vi "DblMonoPMDCurrentScanSM correction.vi"() -> ()   [LabVIEW 2010]
uses:
  <vilib>/DAQmx/write.llb/DAQmx Write (Analog DBL 1Chan 1Samp).vi
  <vilib>/DAQmx/read.llb/DAQmx Read (Analog 1D DBL 1Chan NSamp).vi
  <vilib>/DAQmx/read.llb/DAQmx Read (Analog 1D DBL NChan 1Samp).vi
  <vilib>/DAQmx/write.llb/DAQmx Write (Analog 2D DBL NChan NSamp).vi
  <vilib>/DAQmx/create/channels.llb/DAQmx Create Channel (AO-Voltage-Basic).vi
  <vilib>/DAQmx/create/channels.llb/DAQmx Create Channel (AI-Voltage-Basic).vi
  <vilib>/daqmx/miscellaneous.llb/DAQmx Fill In Error Info.vi
  <vilib>/DAQmx/configure/timing.llb/DAQmx Timing (Sample Clock).vi
  <vilib>/Utility/file.llb/Write To Spreadsheet File (DBL).vi
  <vilib>/Analysis/NI_AALBase.lvlib
panel:
  out "element 2":dbl=0.021735275146704158
  out "element":dbl=0.029564787036695163
  out "number of samples written per channel":u32=999
  out "Waveform Chart  Y":dbl[](graph)=[0.022057757713531734, 0.02205806778326472, 0.022058377852997708, 0.022058687922730698, 0.022058997992463684, 0.02205930806219667, 0.022059618131929658, 0.022059928201662644, 0.022060238271395635, 0.02206054834112862, 0.022060858410861608, 0.022061168480594594, 0.02206147855032758, 0.02206178862006057, 0.022062098689793558, 0.022062408759526544, 0.02206271882925953, 0.022063028898992518, 0.022063338968725504, 0.022063649038458494, 0.02206395910819148, 0.022064269177924468, 0.022064579247657454, 0.02206488931739044, 0.02206519938712343, 0.022065509456856418, 0.022065819526589404, 0.02206612959632239, 0.022066439666055378, 0.022066749735788368, 0.022067059805521354, 0.02206736987525434, 0.022067679944987328, 0.022067990014720314, 0.022068300084453304, 0.02206861015418629, 0.022068920223919278, 0.022069230293652264, 0.02206954036338525, 0.022069850433118238, 0.022070160502851228, 0.022070470572584214, 0.0220707806423172, 0.022071090712050188, 0.022071400781783174, 0.022071710851516164, 0.02207202092124915, 0.022072330990982138, 0.022072641060715124, 0.02207295113044811, 0.0220732612001811, 0.022073571269914088, 0.022073881339647074, 0.02207419140938006, 0.022074501479113048, 0.022074811548846038, 0.022075121618579024, 0.02207543168831201, 0.022075741758044998, 0.022076051827777984, 0.022076361897510974, 0.02207667196724396, 0.022076982036976948, 0.022077292106709934, 0.02207760217644292, 0.022077912246175908, 0.022078222315908898, 0.022078532385641884, 0.02207884245537487, 0.022079152525107858, 0.022079462594840844, 0.022079772664573834, 0.02208008273430682, 0.022080392804039808, 0.022080702873772794, 0.02208101294350578, 0.02208132301323877, 0.022081633082971758, 0.022081943152704744, 0.02208225322243773, 0.022082563292170718, 0.022082873361903708, 0.022083183431636694, 0.02208349350136968, 0.022083803571102668, 0.022084113640835654, 0.022084423710568644, 0.02208473378030163, 0.022085043850034618, 0.022085353919767604, 0.02208566398950059, 0.022085974059233578, 0.022086284128966568, 0.022086594198699554, 0.02208690426843254, 0.022087214338165528, 0.022087524407898514, 0.022087834477631504, 0.02208814454736449, 0.022088454617097478, 0.022088764686830464, 0.02208907475656345, 0.02208938482629644, 0.022089694896029428, 0.022090004965762414, 0.0220903150354954, 0.022090625105228388, 0.022090935174961378, 0.022091245244694364, 0.02209155531442735, 0.022091865384160338, 0.022092175453893324, 0.022092485523626314, 0.0220927955933593, 0.022093105663092288, 0.022093415732825274, 0.02209372580255826, 0.022094035872291248, 0.022094345942024238, 0.022094656011757224, 0.02209496608149021, 0.022095276151223198, 0.022095586220956184, 0.022095896290689174, 0.02209620636042216, 0.022096516430155148, 0.022096826499888134, 0.02209713656962112, 0.02209744663935411, 0.022097756709087098, 0.022098066778820084, 0.02209837684855307, 0.022098686918286058, 0.022098996988019048, 0.022099307057752034, 0.02209961712748502, 0.022099927197218008, 0.022100237266950994, 0.022100547336683984, 0.02210085740641697, 0.022101167476149958, 0.022101477545882944, 0.02210178761561593, 0.022102097685348918, 0.022102407755081908, 0.022102717824814894, 0.02210302789454788, 0.022103337964280868, 0.022103648034013854, 0.022103958103746844, 0.02210426817347983, 0.022104578243212818, 0.022104888312945804, 0.02210519838267879, 0.02210550845241178, 0.022105818522144768, 0.022106128591877754, 0.02210643866161074, 0.022106748731343728, 0.022107058801076718, 0.022107368870809704, 0.02210767894054269, 0.022107989010275678, 0.022108299080008664, 0.02210860914974165, 0.02210891921947464, 0.022109229289207628, 0.022109539358940614, 0.0221098494286736, 0.022110159498406588, 0.022110469568139578, 0.022110779637872564, 0.02211108970760555, 0.022111399777338538, 0.022111709847071524, 0.022112019916804514, 0.0221123299865375, 0.022112640056270488, 0.022112950126003474, 0.02211326019573646, 0.02211357026546945, 0.022113880335202438, 0.022114190404935424, 0.02211450047466841, 0.022114810544401398, 0.022115120614134388, 0.022115430683867374, 0.02211574075360036, 0.022116050823333348, 0.022116360893066334, 0.02211667096279932, 0.02211698103253231, 0.022117291102265298, 0.022117601171998284, 0.02211791124173127, 0.022118221311464258, 0.022118531381197248, 0.022118841450930234, 0.02211915152066322, 0.022119461590396208, 0.022119771660129194, 0.022120081729862184, 0.02212039179959517, 0.022120701869328158, 0.022121011939061144, 0.02212132200879413, 0.02212163207852712, 0.022121942148260108, 0.022122252217993094, 0.02212256228772608, 0.022122872357459068, 0.022123182427192058, 0.022123492496925044, 0.02212380256665803, 0.022124112636391018, 0.022124422706124004, 0.02212473277585699, 0.02212504284558998, 0.022125352915322968, 0.022125662985055954, 0.02212597305478894, 0.022126283124521928, 0.022126593194254918, 0.022126903263987904, 0.02212721333372089, 0.022127523403453878, 0.022127833473186864, 0.022128143542919854, 0.02212845361265284, 0.022128763682385828, 0.022129073752118814, 0.0221293838218518, 0.02212969389158479, 0.022130003961317778, 0.022130314031050764, 0.02213062410078375, 0.022130934170516738, 0.022131244240249728, 0.022131554309982714, 0.0221318643797157, 0.022132174449448688, 0.022132484519181674, 0.02213279458891466, 0.02213310465864765, 0.022133414728380638, 0.022133724798113624, 0.02213403486784661, 0.022134344937579598, 0.022134655007312588, 0.022134965077045574, 0.02213527514677856, 0.022135585216511548, 0.022135895286244534, 0.022136205355977524, 0.02213651542571051, 0.022136825495443498, 0.022137135565176484, 0.02213744563490947, 0.02213775570464246, 0.022138065774375448, 0.022138375844108434, 0.02213868591384142, 0.022138995983574408, 0.022139306053307398, 0.022139616123040384, 0.02213992619277337, 0.022140236262506358, 0.022140546332239344, 0.02214085640197233, 0.02214116647170532, 0.022141476541438308, 0.022141786611171294, 0.02214209668090428, 0.022142406750637268, 0.022142716820370258, 0.022143026890103244, 0.02214333695983623, 0.022143647029569218, 0.022143957099302204, 0.022144267169035194, 0.02214457723876818, 0.022144887308501168, 0.022145197378234154, 0.02214550744796714, 0.02214581751770013, 0.022146127587433118, 0.022146437657166104, 0.02214674772689909, 0.022147057796632078, 0.022147367866365064, 0.022147677936098054, 0.02214798800583104, 0.022148298075564028, 0.022148608145297014, 0.02214891821503, 0.02214922828476299, 0.022149538354495978, 0.022149848424228964, 0.02215015849396195, 0.022150468563694937, 0.022150778633427928, 0.022151088703160914, 0.0221513987728939, 0.022151708842626888, 0.022152018912359874, 0.022152328982092864, 0.02215263905182585, 0.022152949121558838, 0.022153259191291824, 0.02215356926102481, 0.0221538793307578, 0.022154189400490788, 0.022154499470223774, 0.02215480953995676, 0.022155119609689748, 0.022155429679422734, 0.022155739749155724, 0.02215604981888871, 0.022156359888621698, 0.022156669958354684, 0.02215698002808767, 0.02215729009782066, 0.022157600167553648, 0.022157910237286634, 0.02215822030701962, 0.022158530376752607, 0.022158840446485598, 0.022159150516218584, 0.02215946058595157, 0.022159770655684558, 0.022160080725417544, 0.022160390795150534, 0.02216070086488352, 0.022161010934616508, 0.022161321004349494, 0.02216163107408248, 0.02216194114381547, 0.022162251213548458, 0.022162561283281444, 0.02216287135301443, 0.022163181422747417, 0.022163491492480404, 0.022163801562213394, 0.02216411163194638, 0.022164421701679368, 0.022164731771412354, 0.02216504184114534, 0.02216535191087833, 0.022165661980611318, 0.022165972050344304, 0.02216628212007729, 0.022166592189810277, 0.022166902259543268, 0.022167212329276254, 0.02216752239900924, 0.022167832468742227, 0.022168142538475214, 0.022168452608208204, 0.02216876267794119, 0.022169072747674178, 0.022169382817407164, 0.02216969288714015, 0.02217000295687314, 0.022170313026606128, 0.022170623096339114, 0.0221709331660721, 0.022171243235805087, 0.022171553305538074, 0.022171863375271064, 0.02217217344500405, 0.022172483514737037, 0.022172793584470024, 0.02217310365420301, 0.022173413723936, 0.022173723793668988, 0.022174033863401974, 0.02217434393313496, 0.022174654002867947, 0.022174964072600938, 0.022175274142333924, 0.02217558421206691, 0.022175894281799897, 0.022176204351532884, 0.022176514421265874, 0.02217682449099886, 0.022177134560731847, 0.022177444630464834, 0.02217775470019782, 0.02217806476993081, 0.022178374839663798, 0.022178684909396784, 0.02217899497912977, 0.022179305048862757, 0.022179615118595744, 0.022179925188328734, 0.02218023525806172, 0.022180545327794707, 0.022180855397527694, 0.02218116546726068, 0.02218147553699367, 0.022181785606726658, 0.022182095676459644, 0.02218240574619263, 0.022182715815925617, 0.022183025885658608, 0.022183335955391594, 0.02218364602512458, 0.022183956094857567, 0.022184266164590554, 0.022184576234323544, 0.02218488630405653, 0.022185196373789517, 0.022185506443522504, 0.02218581651325549, 0.022186126582988477, 0.022186436652721468, 0.022186746722454454, 0.02218705679218744, 0.022187366861920427, 0.022187676931653414, 0.022187987001386404, 0.02218829707111939, 0.022188607140852377, 0.022188917210585364, 0.02218922728031835, 0.02218953735005134, 0.022189847419784327, 0.022190157489517314, 0.0221904675592503, 0.022190777628983287, 0.022191087698716278, 0.022191397768449264, 0.02219170783818225, 0.022192017907915237, 0.022192327977648224, 0.022192638047381214, 0.0221929481171142, 0.022193258186847187, 0.022193568256580174, 0.02219387832631316, 0.022194188396046147, 0.022194498465779137, 0.022194808535512124, 0.02219511860524511, 0.022195428674978097, 0.022195738744711084, 0.022196048814444074, 0.02219635888417706, 0.022196668953910047, 0.022196979023643034, 0.02219728909337602, 0.02219759916310901, 0.022197909232841997, 0.022198219302574984, 0.02219852937230797, 0.022198839442040957, 0.022199149511773947, 0.022199459581506934, 0.02219976965123992, 0.022200079720972907, 0.022200389790705894, 0.022200699860438884, 0.02220100993017187, 0.022201319999904857, 0.022201630069637844, 0.02220194013937083, 0.022202250209103817, 0.022202560278836807, 0.022202870348569794, 0.02220318041830278, 0.022203490488035767, 0.022203800557768754, 0.022204110627501744, 0.02220442069723473, 0.022204730766967717, 0.022205040836700704, 0.02220535090643369, 0.02220566097616668, 0.022205971045899667, 0.022206281115632654, 0.02220659118536564, 0.022206901255098627, 0.022207211324831617, 0.022207521394564604, 0.02220783146429759, 0.022208141534030577, 0.022208451603763564, 0.022208761673496554, 0.02220907174322954, 0.022209381812962527, 0.022209691882695514, 0.0222100019524285, 0.022210312022161487, 0.022210622091894477, 0.022210932161627464, 0.02221124223136045, 0.022211552301093437, 0.022211862370826424, 0.022212172440559414, 0.0222124825102924, 0.022212792580025387, 0.022213102649758374, 0.02221341271949136, 0.02221372278922435, 0.022214032858957337, 0.022214342928690324, 0.02221465299842331, 0.022214963068156297, 0.022215273137889287, 0.022215583207622274, 0.02221589327735526, 0.022216203347088247, 0.022216513416821234, 0.02221682348655422, 0.02221713355628721, 0.022217443626020197, 0.022217753695753184, 0.02221806376548617, 0.022218373835219157, 0.022218683904952147, 0.022218993974685134, 0.02221930404441812, 0.022219614114151107, 0.022219924183884094, 0.022220234253617084, 0.02222054432335007, 0.022220854393083057, 0.022221164462816044, 0.02222147453254903, 0.02222178460228202, 0.022222094672015007, 0.022222404741747994, 0.02222271481148098, 0.022223024881213967, 0.022223334950946957, 0.022223645020679944, 0.02222395509041293, 0.022224265160145917, 0.022224575229878904, 0.02222488529961189, 0.02222519536934488, 0.022225505439077867, 0.022225815508810854, 0.02222612557854384, 0.022226435648276827, 0.022226745718009817, 0.022227055787742804, 0.02222736585747579, 0.022227675927208777, 0.022227985996941764, 0.022228296066674754, 0.02222860613640774, 0.022228916206140727, 0.022229226275873714, 0.0222295363456067, 0.02222984641533969, 0.022230156485072677, 0.022230466554805664, 0.02223077662453865, 0.022231086694271637, 0.022231396764004627, 0.022231706833737614, 0.0222320169034706, 0.022232326973203587, 0.022232637042936574, 0.02223294711266956, 0.02223325718240255, 0.022233567252135537, 0.022233877321868524, 0.02223418739160151, 0.022234497461334497, 0.022234807531067487, 0.022235117600800474, 0.02223542767053346, 0.022235737740266447, 0.022236047809999434, 0.022236357879732424, 0.02223666794946541, 0.022236978019198397, 0.022237288088931384, 0.02223759815866437, 0.02223790822839736, 0.022238218298130347, 0.022238528367863334, 0.02223883843759632, 0.022239148507329307, 0.022239458577062297, 0.022239768646795284, 0.02224007871652827, 0.022240388786261257, 0.022240698855994244, 0.02224100892572723, 0.02224131899546022, 0.022241629065193207, 0.022241939134926194, 0.02224224920465918, 0.022242559274392167, 0.022242869344125157, 0.022243179413858144, 0.02224348948359113, 0.022243799553324117, 0.022244109623057104, 0.022244419692790094, 0.02224472976252308, 0.022245039832256067, 0.022245349901989054, 0.02224565997172204, 0.02224597004145503, 0.022246280111188017, 0.022246590180921004, 0.02224690025065399, 0.022247210320386977, 0.022247520390119967, 0.022247830459852954, 0.02224814052958594, 0.022248450599318927, 0.022248760669051914, 0.0222490707387849, 0.02224938080851789, 0.022249690878250877, 0.022250000947983864, 0.02225031101771685, 0.022250621087449837, 0.022250931157182827, 0.022251241226915814, 0.0222515512966488, 0.022251861366381787, 0.022252171436114774, 0.022252481505847764, 0.02225279157558075, 0.022253101645313737, 0.022253411715046724, 0.02225372178477971, 0.0222540318545127, 0.022254341924245687, 0.022254651993978674, 0.02225496206371166, 0.022255272133444647, 0.022255582203177634, 0.022255892272910624, 0.02225620234264361, 0.022256512412376597, 0.022256822482109584, 0.02225713255184257, 0.02225744262157556, 0.022257752691308547, 0.022258062761041534, 0.02225837283077452, 0.022258682900507507, 0.022258992970240497, 0.022259303039973484, 0.02225961310970647, 0.022259923179439457, 0.022260233249172444, 0.022260543318905434, 0.02226085338863842, 0.022261163458371407, 0.022261473528104394, 0.02226178359783738, 0.02226209366757037, 0.022262403737303357, 0.022262713807036344, 0.02226302387676933, 0.022263333946502317, 0.022263644016235304, 0.022263954085968294, 0.02226426415570128, 0.022264574225434267, 0.022264884295167254, 0.02226519436490024, 0.02226550443463323, 0.022265814504366217, 0.022266124574099204, 0.02226643464383219, 0.022266744713565177, 0.022267054783298167, 0.022267364853031154, 0.02226767492276414, 0.022267984992497127, 0.022268295062230114, 0.022268605131963104, 0.02226891520169609, 0.022269225271429077, 0.022269535341162064, 0.02226984541089505, 0.02227015548062804, 0.022270465550361027, 0.022270775620094014, 0.022271085689827, 0.022271395759559987, 0.022271705829292974, 0.022272015899025964, 0.02227232596875895, 0.022272636038491937, 0.022272946108224924, 0.02227325617795791, 0.0222735662476909, 0.022273876317423887, 0.022274186387156874, 0.02227449645688986, 0.022274806526622847, 0.022275116596355837, 0.022275426666088824, 0.02227573673582181, 0.022276046805554797, 0.022276356875287784, 0.022276666945020774, 0.02227697701475376, 0.022277287084486747, 0.022277597154219734, 0.02227790722395272, 0.02227821729368571, 0.022278527363418697, 0.022278837433151684, 0.02227914750288467, 0.022279457572617657, 0.022279767642350644, 0.022280077712083634, 0.02228038778181662, 0.022280697851549607, 0.022281007921282594, 0.02228131799101558, 0.02228162806074857, 0.022281938130481557, 0.022282248200214544, 0.02228255826994753, 0.022282868339680517, 0.022283178409413507, 0.022283488479146494, 0.02228379854887948, 0.022284108618612467, 0.022284418688345454, 0.022284728758078444, 0.02228503882781143, 0.022285348897544417, 0.022285658967277404, 0.02228596903701039, 0.02228627910674338, 0.022286589176476367, 0.022286899246209354, 0.02228720931594234, 0.022287519385675327, 0.022287829455408314, 0.022288139525141304, 0.02228844959487429, 0.022288759664607277, 0.022289069734340264, 0.02228937980407325, 0.02228968987380624, 0.022289999943539227, 0.022290310013272214, 0.0222906200830052, 0.022290930152738187, 0.022291240222471177, 0.022291550292204164, 0.02229186036193715, 0.022292170431670137, 0.022292480501403124, 0.022292790571136114, 0.0222931006408691, 0.022293410710602087, 0.022293720780335074, 0.02229403085006806, 0.02229434091980105, 0.022294650989534037, 0.022294961059267024, 0.02229527112900001, 0.022295581198732997, 0.022295891268465984, 0.022296201338198974, 0.02229651140793196, 0.022296821477664947, 0.022297131547397934, 0.02229744161713092, 0.02229775168686391, 0.022298061756596897, 0.022298371826329884, 0.02229868189606287, 0.022298991965795857, 0.022299302035528847, 0.022299612105261834, 0.02229992217499482, 0.022300232244727807, 0.022300542314460794, 0.022300852384193784, 0.02230116245392677, 0.022301472523659757, 0.022301782593392744, 0.02230209266312573, 0.022302402732858717, 0.022302712802591707, 0.022303022872324694, 0.02230333294205768, 0.022303643011790667, 0.022303953081523654, 0.022304263151256644, 0.02230457322098963, 0.022304883290722617, 0.022305193360455604, 0.02230550343018859, 0.02230581349992158, 0.022306123569654567, 0.022306433639387554, 0.02230674370912054, 0.022307053778853527, 0.022307363848586517, 0.022307673918319504, 0.02230798398805249, 0.022308294057785477, 0.022308604127518464, 0.022308914197251454, 0.02230922426698444, 0.022309534336717427, 0.022309844406450414, 0.0223101544761834, 0.022310464545916387, 0.022310774615649377, 0.022311084685382364, 0.02231139475511535, 0.022311704824848337, 0.022312014894581324, 0.022312324964314314, 0.0223126350340473, 0.022312945103780287, 0.022313255173513274, 0.02231356524324626, 0.02231387531297925, 0.022314185382712237, 0.022314495452445224, 0.02231480552217821, 0.022315115591911197, 0.022315425661644187, 0.022315735731377174, 0.02231604580111016, 0.022316355870843147, 0.022316665940576134, 0.022316976010309124, 0.02231728608004211, 0.022317596149775097, 0.022317906219508084, 0.02231821628924107, 0.022318526358974057, 0.022318836428707047, 0.022319146498440034, 0.02231945656817302, 0.022319766637906007, 0.022320076707638994, 0.022320386777371984, 0.02232069684710497, 0.022321006916837957, 0.022321316986570944, 0.02232162705630393, 0.02232193712603692, 0.022322247195769907, 0.022322557265502894, 0.02232286733523588, 0.022323177404968867, 0.022323487474701857, 0.022323797544434844, 0.02232410761416783, 0.022324417683900817, 0.022324727753633804, 0.022325037823366794, 0.02232534789309978, 0.022325657962832767, 0.022325968032565754, 0.02232627810229874, 0.022326588172031727, 0.022326898241764717, 0.022327208311497704, 0.02232751838123069, 0.022327828450963677, 0.022328138520696664, 0.022328448590429654, 0.02232875866016264, 0.022329068729895627, 0.022329378799628614, 0.0223296888693616, 0.02232999893909459, 0.022330309008827577, 0.022330619078560564, 0.02233092914829355, 0.022331239218026537, 0.022331549287759527, 0.022331859357492514, 0.0223321694272255, 0.022332479496958487, 0.022332789566691474, 0.022333099636424464, 0.02233340970615745, 0.022333719775890437, 0.022334029845623424, 0.02233433991535641, 0.022334649985089397, 0.022334960054822387, 0.022335270124555374, 0.02233558019428836, 0.022335890264021347, 0.022336200333754334, 0.022336510403487324, 0.02233682047322031, 0.022337130542953297, 0.022337440612686284, 0.02233775068241927, 0.02233806075215226, 0.022338370821885247, 0.022338680891618234, 0.02233899096135122, 0.022339301031084207, 0.022339611100817197, 0.022339921170550184, 0.02234023124028317, 0.022340541310016157, 0.022340851379749144, 0.02234116144948213, 0.02234147151921512, 0.022341781588948107, 0.022342091658681094, 0.02234240172841408, 0.022342711798147067, 0.022343021867880057, 0.022343331937613044, 0.02234364200734603, 0.022343952077079017, 0.022344262146812004, 0.022344572216544994, 0.02234488228627798, 0.022345192356010967, 0.022345502425743954, 0.02234581249547694, 0.02234612256520993, 0.022346432634942917, 0.022346742704675904, 0.02234705277440889, 0.022347362844141877, 0.022347672913874867, 0.022347982983607854, 0.02234829305334084, 0.022348603123073827, 0.022348913192806814, 0.0223492232625398, 0.02234953333227279, 0.022349843402005777, 0.022350153471738764, 0.02235046354147175, 0.022350773611204737, 0.022351083680937727, 0.022351393750670714, 0.0223517038204037, 0.022352013890136687, 0.022352323959869674, 0.022352634029602664, 0.02235294409933565, 0.022353254169068637, 0.022353564238801624, 0.02235387430853461, 0.0223541843782676, 0.022354494448000587, 0.022354804517733574, 0.02235511458746656, 0.022355424657199547, 0.022355734726932537, 0.022356044796665524, 0.02235635486639851, 0.022356664936131497, 0.022356975005864484, 0.02235728507559747, 0.02235759514533046, 0.022357905215063447, 0.022358215284796434, 0.02235852535452942, 0.022358835424262407, 0.022359145493995397, 0.022359455563728384, 0.02235976563346137, 0.022360075703194357, 0.022360385772927344, 0.022360695842660334, 0.02236100591239332, 0.022361315982126307, 0.022361626051859294, 0.02236193612159228, 0.02236224619132527, 0.022362556261058257, 0.022362866330791244, 0.02236317640052423, 0.022363486470257217, 0.022363796539990207, 0.022364106609723194, 0.02236441667945618, 0.022364726749189167, 0.022365036818922154, 0.02236534688865514, 0.02236565695838813, 0.022365967028121117, 0.022366277097854104, 0.02236658716758709, 0.022366897237320077, 0.022367207307053067, 0.022367517376786054]
  out "initial y":dbl=0.022057757713531734
  out "Final Y":dbl=0.022367517376786054
  out "Waveform Chart X":dbl[](graph)=[0.030209752173193244, 0.030210266929154354, 0.030210781685115463, 0.030211296441076577, 0.030211811197037686, 0.030212325952998796, 0.03021284070895991, 0.03021335546492102, 0.03021387022088213, 0.030214384976843242, 0.030214899732804352, 0.03021541448876546, 0.030215929244726575, 0.030216444000687685, 0.030216958756648794, 0.030217473512609908, 0.030217988268571017, 0.03021850302453213, 0.03021901778049324, 0.03021953253645435, 0.030220047292415463, 0.030220562048376573, 0.030221076804337683, 0.030221591560298796, 0.030222106316259906, 0.030222621072221015, 0.03022313582818213, 0.03022365058414324, 0.03022416534010435, 0.03022468009606546, 0.03022519485202657, 0.030225709607987684, 0.030226224363948794, 0.030226739119909904, 0.030227253875871017, 0.030227768631832127, 0.030228283387793237, 0.03022879814375435, 0.03022931289971546, 0.03022982765567657, 0.030230342411637683, 0.030230857167598792, 0.030231371923559902, 0.030231886679521015, 0.030232401435482125, 0.03023291619144324, 0.030233430947404348, 0.030233945703365458, 0.03023446045932657, 0.03023497521528768, 0.03023548997124879, 0.030236004727209904, 0.030236519483171014, 0.030237034239132123, 0.030237548995093236, 0.030238063751054346, 0.030238578507015456, 0.03023909326297657, 0.03023960801893768, 0.030240122774898792, 0.030240637530859902, 0.03024115228682101, 0.030241667042782125, 0.030242181798743235, 0.030242696554704344, 0.030243211310665458, 0.030243726066626567, 0.030244240822587677, 0.03024475557854879, 0.0302452703345099, 0.03024578509047101, 0.030246299846432123, 0.030246814602393233, 0.030247329358354346, 0.030247844114315456, 0.030248358870276566, 0.03024887362623768, 0.03024938838219879, 0.0302499031381599, 0.03025041789412101, 0.03025093265008212, 0.03025144740604323, 0.030251962162004344, 0.030252476917965454, 0.030252991673926564, 0.030253506429887677, 0.030254021185848787, 0.0302545359418099, 0.03025505069777101, 0.03025556545373212, 0.030256080209693233, 0.030256594965654342, 0.030257109721615452, 0.030257624477576565, 0.030258139233537675, 0.030258653989498785, 0.030259168745459898, 0.030259683501421008, 0.030260198257382118, 0.03026071301334323, 0.03026122776930434, 0.030261742525265454, 0.030262257281226564, 0.030262772037187673, 0.030263286793148787, 0.030263801549109896, 0.030264316305071006, 0.03026483106103212, 0.03026534581699323, 0.03026586057295434, 0.030266375328915452, 0.030266890084876562, 0.03026740484083767, 0.030267919596798785, 0.030268434352759895, 0.030268949108721008, 0.030269463864682117, 0.030269978620643227, 0.03027049337660434, 0.03027100813256545, 0.03027152288852656, 0.030272037644487673, 0.030272552400448783, 0.030273067156409893, 0.030273581912371006, 0.030274096668332116, 0.030274611424293225, 0.03027512618025434, 0.03027564093621545, 0.03027615569217656, 0.03027667044813767, 0.03027718520409878, 0.030277699960059894, 0.030278214716021004, 0.030278729471982114, 0.030279244227943227, 0.030279758983904337, 0.030280273739865447, 0.03028078849582656, 0.03028130325178767, 0.03028181800774878, 0.030282332763709893, 0.030282847519671002, 0.030283362275632116, 0.030283877031593225, 0.030284391787554335, 0.030284906543515448, 0.030285421299476558, 0.030285936055437668, 0.03028645081139878, 0.03028696556735989, 0.030287480323321, 0.030287995079282114, 0.030288509835243223, 0.030289024591204333, 0.030289539347165446, 0.030290054103126556, 0.03029056885908767, 0.03029108361504878, 0.03029159837100989, 0.030292113126971002, 0.030292627882932112, 0.03029314263889322, 0.030293657394854335, 0.030294172150815445, 0.030294686906776554, 0.030295201662737668, 0.030295716418698777, 0.030296231174659887, 0.030296745930621, 0.03029726068658211, 0.030297775442543223, 0.030298290198504333, 0.030298804954465443, 0.030299319710426556, 0.030299834466387666, 0.030300349222348776, 0.03030086397830989, 0.030301378734271, 0.030301893490232108, 0.03030240824619322, 0.03030292300215433, 0.03030343775811544, 0.030303952514076554, 0.030304467270037664, 0.030304982025998777, 0.030305496781959887, 0.030306011537920997, 0.03030652629388211, 0.03030704104984322, 0.03030755580580433, 0.030308070561765443, 0.030308585317726552, 0.030309100073687662, 0.030309614829648775, 0.030310129585609885, 0.030310644341570995, 0.030311159097532108, 0.030311673853493218, 0.03031218860945433, 0.03031270336541544, 0.03031321812137655, 0.030313732877337664, 0.030314247633298774, 0.030314762389259883, 0.030315277145220997, 0.030315791901182106, 0.030316306657143216, 0.03031682141310433, 0.03031733616906544, 0.03031785092502655, 0.030318365680987662, 0.030318880436948772, 0.030319395192909885, 0.030319909948870995, 0.030320424704832104, 0.030320939460793218, 0.030321454216754327, 0.030321968972715437, 0.03032248372867655, 0.03032299848463766, 0.03032351324059877, 0.030324027996559883, 0.030324542752520993, 0.030325057508482103, 0.030325572264443216, 0.030326087020404326, 0.03032660177636544, 0.03032711653232655, 0.03032763128828766, 0.03032814604424877, 0.03032866080020988, 0.03032917555617099, 0.030329690312132104, 0.030330205068093214, 0.030330719824054324, 0.030331234580015437, 0.030331749335976547, 0.030332264091937657, 0.03033277884789877, 0.03033329360385988, 0.030333808359820993, 0.030334323115782102, 0.030334837871743212, 0.030335352627704325, 0.030335867383665435, 0.030336382139626545, 0.030336896895587658, 0.030337411651548768, 0.030337926407509878, 0.03033844116347099, 0.0303389559194321, 0.03033947067539321, 0.030339985431354324, 0.030340500187315433, 0.030341014943276547, 0.030341529699237656, 0.030342044455198766, 0.03034255921115988, 0.03034307396712099, 0.0303435887230821, 0.030344103479043212, 0.030344618235004322, 0.03034513299096543, 0.030345647746926545, 0.030346162502887655, 0.030346677258848764, 0.030347192014809878, 0.030347706770770987, 0.0303482215267321, 0.03034873628269321, 0.03034925103865432, 0.030349765794615433, 0.030350280550576543, 0.030350795306537653, 0.030351310062498766, 0.030351824818459876, 0.030352339574420985, 0.0303528543303821, 0.03035336908634321, 0.030353883842304318, 0.03035439859826543, 0.03035491335422654, 0.030355428110187654, 0.030355942866148764, 0.030356457622109874, 0.030356972378070987, 0.030357487134032097, 0.030358001889993207, 0.03035851664595432, 0.03035903140191543, 0.03035954615787654, 0.030360060913837653, 0.030360575669798762, 0.030361090425759872, 0.030361605181720985, 0.030362119937682095, 0.03036263469364321, 0.030363149449604318, 0.030363664205565428, 0.03036417896152654, 0.03036469371748765, 0.03036520847344876, 0.030365723229409874, 0.030366237985370984, 0.030366752741332093, 0.030367267497293206, 0.030367782253254316, 0.030368297009215426, 0.03036881176517654, 0.03036932652113765, 0.030369841277098762, 0.030370356033059872, 0.03037087078902098, 0.030371385544982095, 0.030371900300943205, 0.030372415056904314, 0.030372929812865428, 0.030373444568826537, 0.030373959324787647, 0.03037447408074876, 0.03037498883670987, 0.03037550359267098, 0.030376018348632093, 0.030376533104593203, 0.030377047860554316, 0.030377562616515426, 0.030378077372476536, 0.03037859212843765, 0.03037910688439876, 0.03037962164035987, 0.03038013639632098, 0.03038065115228209, 0.0303811659082432, 0.030381680664204314, 0.030382195420165424, 0.030382710176126534, 0.030383224932087647, 0.030383739688048757, 0.03038425444400987, 0.03038476919997098, 0.03038528395593209, 0.030385798711893203, 0.030386313467854312, 0.030386828223815422, 0.030387342979776535, 0.030387857735737645, 0.030388372491698755, 0.030388887247659868, 0.030389402003620978, 0.030389916759582088, 0.0303904315155432, 0.03039094627150431, 0.030391461027465424, 0.030391975783426534, 0.030392490539387643, 0.030393005295348757, 0.030393520051309866, 0.030394034807270976, 0.03039454956323209, 0.0303950643191932, 0.03039557907515431, 0.030396093831115422, 0.030396608587076532, 0.03039712334303764, 0.030397638098998755, 0.030398152854959865, 0.030398667610920978, 0.030399182366882087, 0.030399697122843197, 0.03040021187880431, 0.03040072663476542, 0.03040124139072653, 0.030401756146687643, 0.030402270902648753, 0.030402785658609863, 0.030403300414570976, 0.030403815170532086, 0.030404329926493195, 0.03040484468245431, 0.03040535943841542, 0.03040587419437653, 0.03040638895033764, 0.03040690370629875, 0.030407418462259864, 0.030407933218220974, 0.030408447974182084, 0.030408962730143197, 0.030409477486104307, 0.030409992242065417, 0.03041050699802653, 0.03041102175398764, 0.03041153650994875, 0.030412051265909863, 0.030412566021870972, 0.030413080777832086, 0.030413595533793195, 0.030414110289754305, 0.030414625045715418, 0.030415139801676528, 0.030415654557637638, 0.03041616931359875, 0.03041668406955986, 0.03041719882552097, 0.030417713581482084, 0.030418228337443193, 0.030418743093404303, 0.030419257849365416, 0.030419772605326526, 0.03042028736128764, 0.03042080211724875, 0.03042131687320986, 0.030421831629170972, 0.030422346385132082, 0.03042286114109319, 0.030423375897054305, 0.030423890653015415, 0.030424405408976524, 0.030424920164937638, 0.030425434920898747, 0.030425949676859857, 0.03042646443282097, 0.03042697918878208, 0.030427493944743193, 0.030428008700704303, 0.030428523456665413, 0.030429038212626526, 0.030429552968587636, 0.030430067724548746, 0.03043058248050986, 0.03043109723647097, 0.030431611992432078, 0.03043212674839319, 0.0304326415043543, 0.03043315626031541, 0.030433671016276524, 0.030434185772237634, 0.030434700528198747, 0.030435215284159857, 0.030435730040120967, 0.03043624479608208, 0.03043675955204319, 0.0304372743080043, 0.030437789063965413, 0.030438303819926522, 0.030438818575887632, 0.030439333331848745, 0.030439848087809855, 0.030440362843770965, 0.030440877599732078, 0.030441392355693188, 0.0304419071116543, 0.03044242186761541, 0.03044293662357652, 0.030443451379537634, 0.030443966135498744, 0.030444480891459853, 0.030444995647420967, 0.030445510403382076, 0.030446025159343186, 0.0304465399153043, 0.03044705467126541, 0.03044756942722652, 0.030448084183187632, 0.030448598939148742, 0.030449113695109855, 0.030449628451070965, 0.030450143207032074, 0.030450657962993188, 0.030451172718954297, 0.030451687474915407, 0.03045220223087652, 0.03045271698683763, 0.03045323174279874, 0.030453746498759853, 0.030454261254720963, 0.030454776010682073, 0.030455290766643186, 0.030455805522604296, 0.03045632027856541, 0.03045683503452652, 0.03045734979048763, 0.03045786454644874, 0.03045837930240985, 0.03045889405837096, 0.030459408814332074, 0.030459923570293184, 0.030460438326254294, 0.030460953082215407, 0.030461467838176517, 0.030461982594137627, 0.03046249735009874, 0.03046301210605985, 0.030463526862020963, 0.030464041617982072, 0.030464556373943182, 0.030465071129904295, 0.030465585885865405, 0.030466100641826515, 0.030466615397787628, 0.030467130153748738, 0.030467644909709848, 0.03046815966567096, 0.03046867442163207, 0.03046918917759318, 0.030469703933554294, 0.030470218689515403, 0.030470733445476513, 0.030471248201437626, 0.030471762957398736, 0.03047227771335985, 0.03047279246932096, 0.03047330722528207, 0.030473821981243182, 0.030474336737204292, 0.0304748514931654, 0.030475366249126515, 0.030475881005087625, 0.030476395761048734, 0.030476910517009848, 0.030477425272970957, 0.030477940028932067, 0.03047845478489318, 0.03047896954085429, 0.030479484296815403, 0.030479999052776513, 0.030480513808737623, 0.030481028564698736, 0.030481543320659846, 0.030482058076620955, 0.03048257283258207, 0.03048308758854318, 0.030483602344504288, 0.0304841171004654, 0.03048463185642651, 0.030485146612387624, 0.030485661368348734, 0.030486176124309844, 0.030486690880270957, 0.030487205636232067, 0.030487720392193177, 0.03048823514815429, 0.0304887499041154, 0.03048926466007651, 0.030489779416037623, 0.030490294171998732, 0.030490808927959842, 0.030491323683920955, 0.030491838439882065, 0.030492353195843175, 0.030492867951804288, 0.030493382707765398, 0.03049389746372651, 0.03049441221968762, 0.03049492697564873, 0.030495441731609844, 0.030495956487570954, 0.030496471243532063, 0.030496985999493176, 0.030497500755454286, 0.030498015511415396, 0.03049853026737651, 0.03049904502333762, 0.03049955977929873, 0.030500074535259842, 0.03050058929122095, 0.030501104047182065, 0.030501618803143175, 0.030502133559104284, 0.030502648315065398, 0.030503163071026507, 0.030503677826987617, 0.03050419258294873, 0.03050470733890984, 0.03050522209487095, 0.030505736850832063, 0.030506251606793173, 0.030506766362754283, 0.030507281118715396, 0.030507795874676506, 0.03050831063063762, 0.03050882538659873, 0.03050934014255984, 0.03050985489852095, 0.03051036965448206, 0.03051088441044317, 0.030511399166404284, 0.030511913922365394, 0.030512428678326504, 0.030512943434287617, 0.030513458190248727, 0.030513972946209836, 0.03051448770217095, 0.03051500245813206, 0.030515517214093173, 0.030516031970054282, 0.030516546726015392, 0.030517061481976505, 0.030517576237937615, 0.030518090993898725, 0.030518605749859838, 0.030519120505820948, 0.030519635261782058, 0.03052015001774317, 0.03052066477370428, 0.03052117952966539, 0.030521694285626504, 0.030522209041587613, 0.030522723797548727, 0.030523238553509836, 0.030523753309470946, 0.03052426806543206, 0.03052478282139317, 0.03052529757735428, 0.030525812333315392, 0.030526327089276502, 0.03052684184523761, 0.030527356601198725, 0.030527871357159835, 0.030528386113120944, 0.030528900869082057, 0.030529415625043167, 0.03052993038100428, 0.03053044513696539, 0.0305309598929265, 0.030531474648887613, 0.030531989404848723, 0.030532504160809833, 0.030533018916770946, 0.030533533672732056, 0.030534048428693165, 0.03053456318465428, 0.03053507794061539, 0.030535592696576498, 0.03053610745253761, 0.03053662220849872, 0.030537136964459834, 0.030537651720420944, 0.030538166476382054, 0.030538681232343167, 0.030539195988304277, 0.030539710744265387, 0.0305402255002265, 0.03054074025618761, 0.03054125501214872, 0.030541769768109833, 0.030542284524070942, 0.030542799280032052, 0.030543314035993165, 0.030543828791954275, 0.030544343547915388, 0.030544858303876498, 0.030545373059837608, 0.03054588781579872, 0.03054640257175983, 0.03054691732772094, 0.030547432083682054, 0.030547946839643163, 0.030548461595604273, 0.030548976351565386, 0.030549491107526496, 0.030550005863487606, 0.03055052061944872, 0.03055103537540983, 0.030551550131370942, 0.030552064887332052, 0.03055257964329316, 0.030553094399254275, 0.030553609155215385, 0.030554123911176494, 0.030554638667137608, 0.030555153423098717, 0.030555668179059827, 0.03055618293502094, 0.03055669769098205, 0.03055721244694316, 0.030557727202904273, 0.030558241958865383, 0.030558756714826496, 0.030559271470787606, 0.030559786226748716, 0.03056030098270983, 0.03056081573867094, 0.030561330494632048, 0.03056184525059316, 0.03056236000655427, 0.03056287476251538, 0.030563389518476494, 0.030563904274437604, 0.030564419030398714, 0.030564933786359827, 0.030565448542320937, 0.03056596329828205, 0.03056647805424316, 0.03056699281020427, 0.030567507566165383, 0.030568022322126492, 0.030568537078087602, 0.030569051834048715, 0.030569566590009825, 0.030570081345970935, 0.030570596101932048, 0.030571110857893158, 0.030571625613854268, 0.03057214036981538, 0.03057265512577649, 0.030573169881737604, 0.030573684637698714, 0.030574199393659823, 0.030574714149620937, 0.030575228905582046, 0.030575743661543156, 0.03057625841750427, 0.03057677317346538, 0.03057728792942649, 0.030577802685387602, 0.030578317441348712, 0.03057883219730982, 0.030579346953270935, 0.030579861709232044, 0.030580376465193158, 0.030580891221154267, 0.030581405977115377, 0.03058192073307649, 0.0305824354890376, 0.03058295024499871, 0.030583465000959823, 0.030583979756920933, 0.030584494512882043, 0.030585009268843156, 0.030585524024804266, 0.030586038780765375, 0.03058655353672649, 0.0305870682926876, 0.03058758304864871, 0.03058809780460982, 0.03058861256057093, 0.030589127316532044, 0.030589642072493154, 0.030590156828454264, 0.030590671584415377, 0.030591186340376487, 0.030591701096337597, 0.03059221585229871, 0.03059273060825982, 0.03059324536422093, 0.030593760120182042, 0.030594274876143152, 0.030594789632104265, 0.030595304388065375, 0.030595819144026485, 0.030596333899987598, 0.030596848655948708, 0.030597363411909818, 0.03059787816787093, 0.03059839292383204, 0.03059890767979315, 0.030599422435754264, 0.030599937191715373, 0.030600451947676483, 0.030600966703637596, 0.030601481459598706, 0.03060199621555982, 0.03060251097152093, 0.03060302572748204, 0.030603540483443152, 0.030604055239404262, 0.03060456999536537, 0.030605084751326485, 0.030605599507287595, 0.030606114263248704, 0.030606629019209818, 0.030607143775170927, 0.030607658531132037, 0.03060817328709315, 0.03060868804305426, 0.030609202799015373, 0.030609717554976483, 0.030610232310937593, 0.030610747066898706, 0.030611261822859816, 0.030611776578820925, 0.03061229133478204, 0.03061280609074315, 0.030613320846704258, 0.03061383560266537, 0.03061435035862648, 0.03061486511458759, 0.030615379870548704, 0.030615894626509814, 0.030616409382470927, 0.030616924138432037, 0.030617438894393147, 0.03061795365035426, 0.03061846840631537, 0.03061898316227648, 0.030619497918237593, 0.030620012674198702, 0.030620527430159812, 0.030621042186120925, 0.030621556942082035, 0.030622071698043145, 0.030622586454004258, 0.030623101209965368, 0.03062361596592648, 0.03062413072188759, 0.0306246454778487, 0.030625160233809814, 0.030625674989770924, 0.030626189745732033, 0.030626704501693146, 0.030627219257654256, 0.030627734013615366, 0.03062824876957648, 0.03062876352553759, 0.0306292782814987, 0.030629793037459812, 0.03063030779342092, 0.030630822549382035, 0.030631337305343145, 0.030631852061304254, 0.030632366817265368, 0.030632881573226477, 0.030633396329187587, 0.0306339110851487, 0.03063442584110981, 0.03063494059707092, 0.030635455353032033, 0.030635970108993143, 0.030636484864954253, 0.030636999620915366, 0.030637514376876476, 0.03063802913283759, 0.0306385438887987, 0.03063905864475981, 0.03063957340072092, 0.03064008815668203, 0.03064060291264314, 0.030641117668604254, 0.030641632424565364, 0.030642147180526474, 0.030642661936487587, 0.030643176692448697, 0.030643691448409806, 0.03064420620437092, 0.03064472096033203, 0.030645235716293143, 0.030645750472254252, 0.030646265228215362, 0.030646779984176475, 0.030647294740137585, 0.030647809496098695, 0.030648324252059808, 0.030648839008020918, 0.030649353763982028, 0.03064986851994314, 0.03065038327590425, 0.03065089803186536, 0.030651412787826474, 0.030651927543787583, 0.030652442299748697, 0.030652957055709806, 0.030653471811670916, 0.03065398656763203, 0.03065450132359314, 0.03065501607955425, 0.030655530835515362, 0.030656045591476472, 0.03065656034743758, 0.030657075103398695, 0.030657589859359805, 0.030658104615320914, 0.030658619371282027, 0.030659134127243137, 0.03065964888320425, 0.03066016363916536, 0.03066067839512647, 0.030661193151087583, 0.030661707907048693, 0.030662222663009803, 0.030662737418970916, 0.030663252174932026, 0.030663766930893135, 0.03066428168685425, 0.03066479644281536, 0.030665311198776468, 0.03066582595473758, 0.03066634071069869, 0.030666855466659804, 0.030667370222620914, 0.030667884978582024, 0.030668399734543137, 0.030668914490504247, 0.030669429246465357, 0.03066994400242647, 0.03067045875838758, 0.03067097351434869, 0.030671488270309803, 0.030672003026270912, 0.030672517782232022, 0.030673032538193135, 0.030673547294154245, 0.030674062050115358, 0.030674576806076468, 0.030675091562037578, 0.03067560631799869, 0.0306761210739598, 0.03067663582992091, 0.030677150585882024, 0.030677665341843133, 0.030678180097804243, 0.030678694853765356, 0.030679209609726466, 0.030679724365687576, 0.03068023912164869, 0.0306807538776098, 0.030681268633570912, 0.030681783389532022, 0.03068229814549313, 0.030682812901454245, 0.030683327657415355, 0.030683842413376464, 0.030684357169337578, 0.030684871925298687, 0.030685386681259797, 0.03068590143722091, 0.03068641619318202, 0.03068693094914313, 0.030687445705104243, 0.030687960461065353, 0.030688475217026463, 0.030688989972987576, 0.030689504728948686, 0.0306900194849098, 0.03069053424087091, 0.030691048996832018, 0.03069156375279313, 0.03069207850875424, 0.03069259326471535, 0.030693108020676464, 0.030693622776637574, 0.030694137532598684, 0.030694652288559797, 0.030695167044520907, 0.03069568180048202, 0.03069619655644313, 0.03069671131240424, 0.030697226068365353, 0.030697740824326462, 0.030698255580287572, 0.030698770336248685, 0.030699285092209795, 0.030699799848170905, 0.030700314604132018, 0.030700829360093128, 0.030701344116054238, 0.03070185887201535, 0.03070237362797646, 0.030702888383937574, 0.030703403139898684, 0.030703917895859793, 0.030704432651820907, 0.030704947407782016, 0.030705462163743126, 0.03070597691970424, 0.03070649167566535, 0.03070700643162646, 0.030707521187587572, 0.030708035943548682, 0.03070855069950979, 0.030709065455470905, 0.030709580211432014, 0.030710094967393124, 0.030710609723354237, 0.030711124479315347, 0.03071163923527646, 0.03071215399123757, 0.03071266874719868, 0.030713183503159793, 0.030713698259120903, 0.030714213015082013, 0.030714727771043126, 0.030715242527004236, 0.030715757282965345, 0.03071627203892646, 0.03071678679488757, 0.03071730155084868, 0.03071781630680979, 0.0307183310627709, 0.030718845818732014, 0.030719360574693124, 0.030719875330654234, 0.030720390086615347, 0.030720904842576457, 0.030721419598537567, 0.03072193435449868, 0.03072244911045979, 0.0307229638664209, 0.030723478622382012, 0.030723993378343122]
  out "initial x":dbl=0.030209752173193244
  out "Final x":dbl=0.030723993378343122
  in  "Volts/pixel":dbl=-0.0002
  out "Xin":dbl=0.030209752173193244
  out "Yin":dbl=0.022057757713531734
  in  "Correction":dbl[][](array[numeric])=[[450.0, 0.0, 0.0], [460.0, 0.0, 0.0], [480.0, 2.0, 1.0], [500.0, 0.0, 2.0], [520.0, -2.0, 3.0], [540.0, -2.0, 2.0], [560.0, -7.0, 4.0], [580.0, -12.0, 4.0], [600.0, -19.0, 6.0], [620.0, -23.0, 7.0], [640.0, -26.0, 8.0], [660.0, -28.0, 9.0], [680.0, -28.0, 9.0], [700.0, -24.0, 8.0], [720.0, -24.0, 8.0], [740.0, -20.0, 8.0], [760.0, -20.0, 8.0], [780.0, -20.0, 8.0]]
  in  "Scan mirrors out":tag="Dev1/ao1:0"
  in  "Scan Mirrors in":tag="Dev1/ai1:2"
  in  "Voltage B":dbl min=-10.0 max=10.0 step=0.1 format="%0.2f"
  in  "Voltage A":dbl min=-10.0 max=10.0 step=0.1 format="%0.2f"
  in  "Output B":tag="Dev1/ao3"
  in  "Output A":tag="Dev1/ao2"
  in  "Input Channel":tag="Dev1/ai18"
  in  "Current":bool=TRUE
  in  "Power":bool
  out "ScanGraph":cluster{dbl[], dbl[]}(graph)={[499.989, 504.988, 509.986, 514.984, 519.999, 524.996, 529.993, 534.99, 539.986, 544.998, 549.994, 554.99, 559.984, 564.995, 569.99, 574.983, 579.993, 584.986, 589.994, 594.986, 599.995, 604.986, 609.993, 614.983, 619.99, 624.995, 629.985, 634.99, 639.994, 644.999, 649.986, 654.989, 659.992, 664.994, 669.996, 674.997, 679.998, 684.998, 689.983, 694.998, 699.997, 704.996, 709.994, 714.991, 719.988, 724.985, 729.997, 734.993, 739.988, 744.999, 749.992, 754.986, 759.996, 764.988, 769.996, 774.987, 779.995, 784.984, 789.991, 794.996, 799.984], [1.2097482190295927, 1.3264473613476158, 1.4110543057909941, 1.54115844941832, 1.7367515094306618, 1.8978866510904335, 1.7264478522708393, 1.8459262312537779, 2.1087680972386513, 2.103954066971629, 2.161514429392974, 2.2109137117937547, 2.2195988324942215, 2.117981766264765, 2.2597296257333013, 2.3844516842269634, 2.5082895200084487, 2.738157407085412, 2.825182521560252, 2.603502453734474, 2.569384986416469, 2.93315974192358, 3.0797470071994617, 3.1192438623439127, 3.164203598063563, 3.0319291055650814, 3.101436625876921, 3.0633664407267016, 2.9351030289000524, 3.148354482020188, 3.072544975547802, 2.9361865742314786, 2.8811953590406842, 2.7956346331410313, 2.9633513158750824, 3.12109201732066, 3.3487395643181523, 3.555959144147924, 3.716572422792752, 3.8172775125024927, 3.7607940533067, 3.5490724944473198, 2.895730344968616, 2.471587998371011, 2.7393789748783575, 3.0100379375623456, 2.9284437396194165, 2.9101795507819537, 3.0200810505695106, 2.880620370566675, 2.840778477171908, 2.7842551524774333, 2.6823600039821414, 2.5155860310944083, 2.296911956087342, 2.034486338500645, 1.8457478975463835, 1.8531337288318512, 2.056709625467515, 2.3600690362392904, 2.513702082576027]}
  in  "Sensitivity":dbl=1.0 caption="(A/V)" format="%#_6p"
  out "Readout":dbl=2.5100277056893323 format="%^#_9e"
  in  "Scan Save Path":path
  in  "On":bool=TRUE
  out "Waveform Chart":dbl(graph)=2.5100277056893323
  in  "Save":bool=TRUE
  in  "Exit":bool
  in  "STOP":bool
  in  "Step Time (sec)":dbl=1.0 min=0.001 max=300.0 step=0.001 format="%.3f"
  in  "Step Size (nm)":dbl=5.0 min=0.1 max=100.0 step=0.1 format="%.1f"
  in  "End":dbl=800.0 min=0.0 max=2000.0 step=0.1 format="%.1f"
  in  "Start":dbl=500.0 min=0.0 max=2000.0 step=0.1 format="%.1f"
  in  "Scan":bool
  in  "Up":bool=TRUE caption="Down"
  in  "Increment (nm)":dbl=10.0 min=0.1 max=2000.0 step=0.1 format="%.1f"
  in  "PMD Settings":T1={"Beam Diameter (mm)"=4.0, "BWIn"=0, "Averaging Rate"=300, "Auto Range"=TRUE} {"Averaging Rate" min=33 max=5000 step=1; "BWIn" items=["HIGH", "LOW"]; "Beam Diameter (mm)" min=1.0 max=9.0 step=0.5}
  in  "Step":bool
  out "Busy":bool
  in  "Send Command":bool
  in  "Command":u16(ring)=1 items=["nm", "goto", "nm/min", "VIS grating", "IR grating"]
  in  "Wavelength (nm)":dbl=800.0 min=0.0 max=2000.0 step=0.1 format="%.1f"
  in  "Scan Speed (nm/min)":dbl=100.0 min=1.0 max=500.0 step=0.1 format="%.1f"
  out "Done?":string="  ok\r\n"
  in  "Send Question":bool
  in  "Ask?":u16(ring) items=["?nm", "?nm/min", "?grating", "?turret", "?gratings"]
  in  "Zero?":bool
  out "PM Error log":string
  out "AUTO?":bool
  out "Zero Value":dbl format="%#.3p"
  out "Rng":string
  in  "Range":i16=1 min=1 max=6 step=1
  in  "Mono Port":refnum<visa-resource-name>="COM11"
  out "IDN String":string="Thorlabs,PM100USB,P2000362,1.3.0\n"
  out "Sensor SN":string="10061433"
  out "Sensor Name":string="S120C"
  out "Reply":string=" 799.984 nm  ok\r\n" caption="Mono Response"
  # "Range Settings"
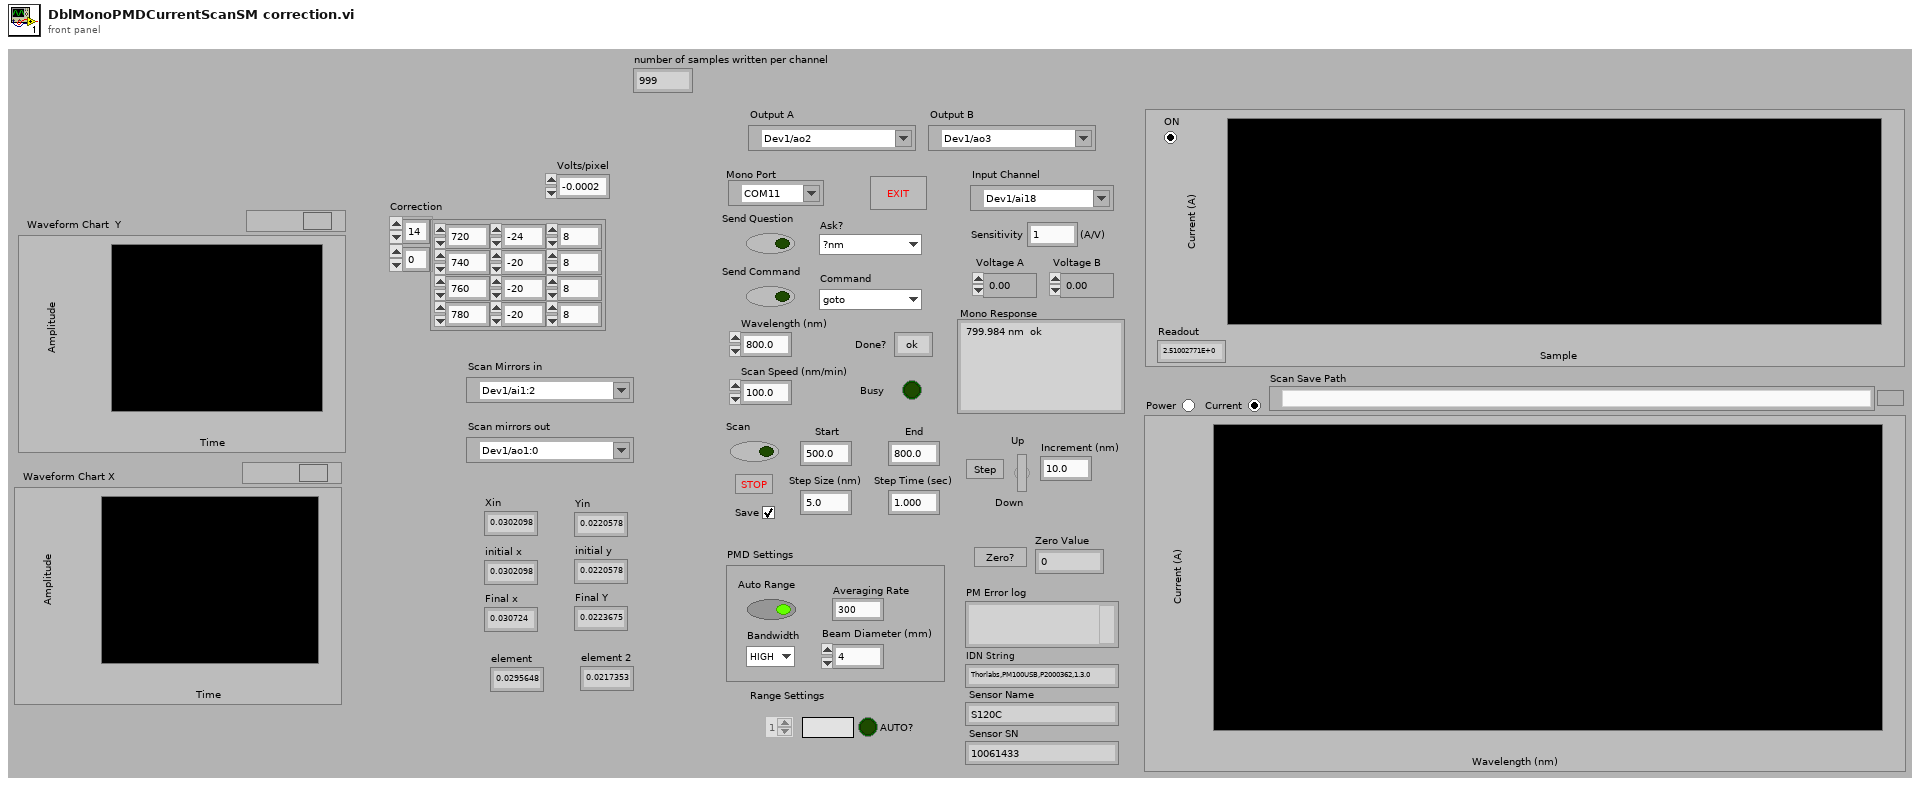
[diagram p1: front panel]
types:
  T1 = cluster{"Beam Diameter (mm)":dbl, "BWIn":u16, "Averaging Rate":i32, "Auto Range":bool}
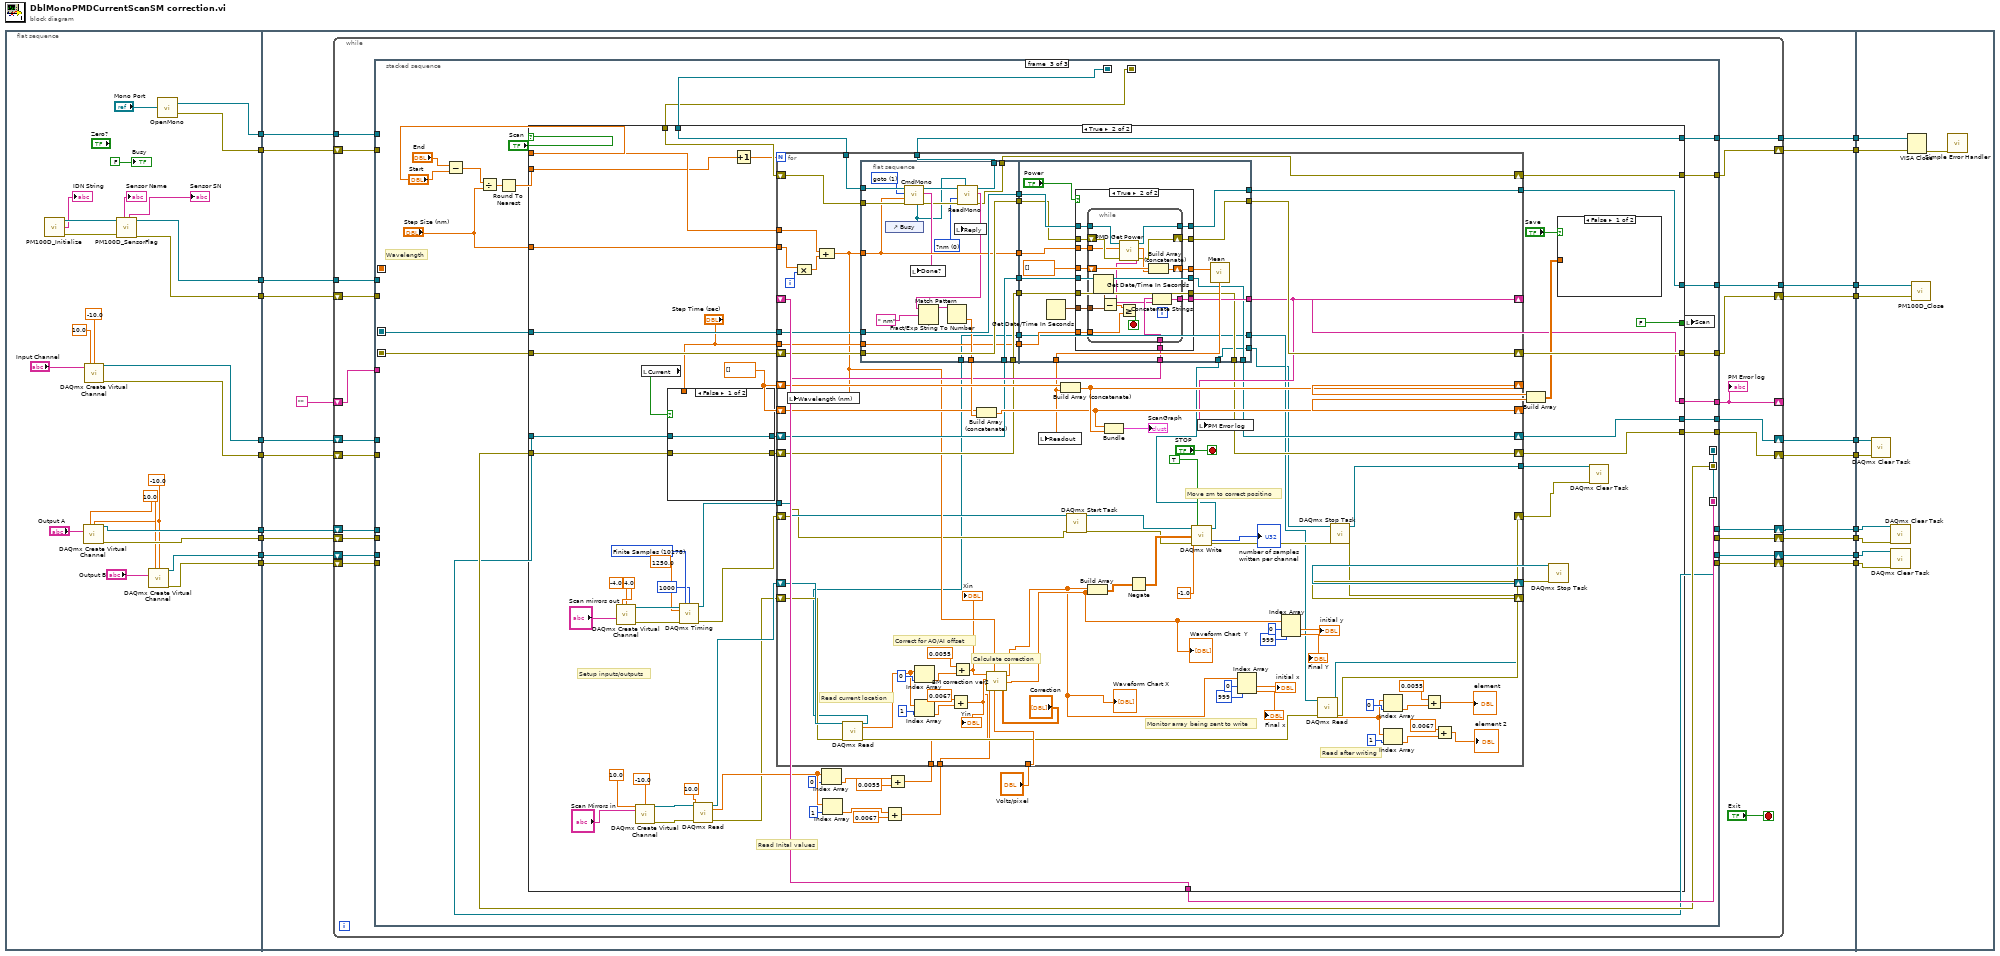
[diagram p0: block diagram]
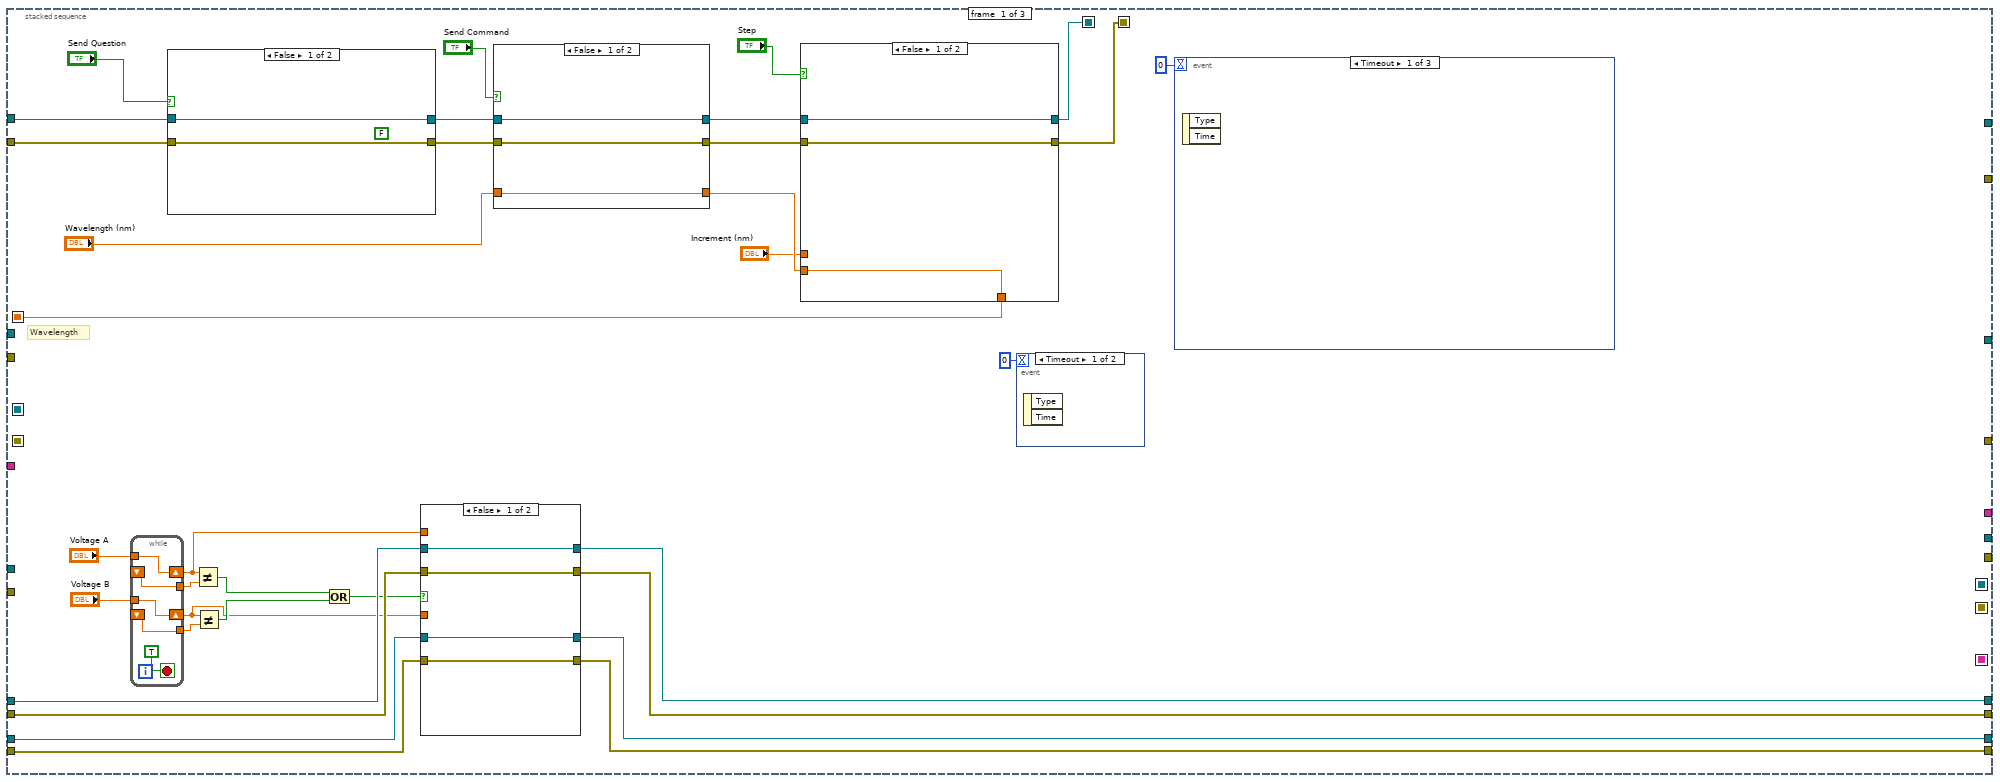
[diagram p2: hidden frame]
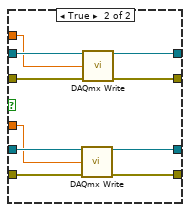
[diagram p3: hidden frame]
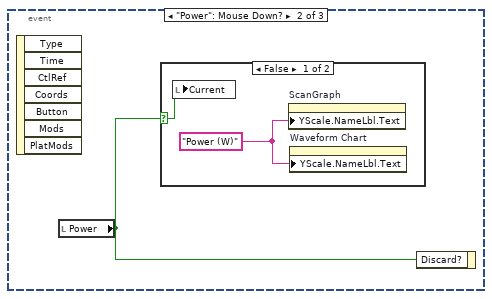
[diagram p4: hidden frame]
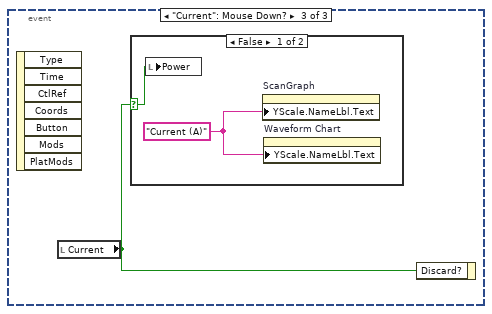
[diagram p6: hidden frame]
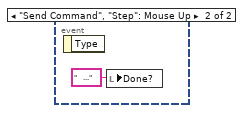
[diagram p8: hidden frame]
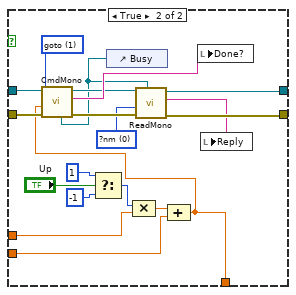
[diagram p9: hidden frame]
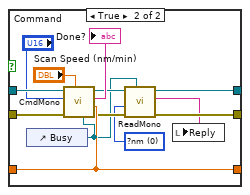
[diagram p10: hidden frame]
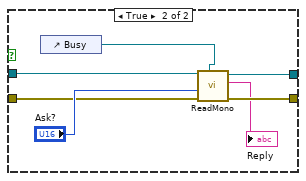
[diagram p11: hidden frame]
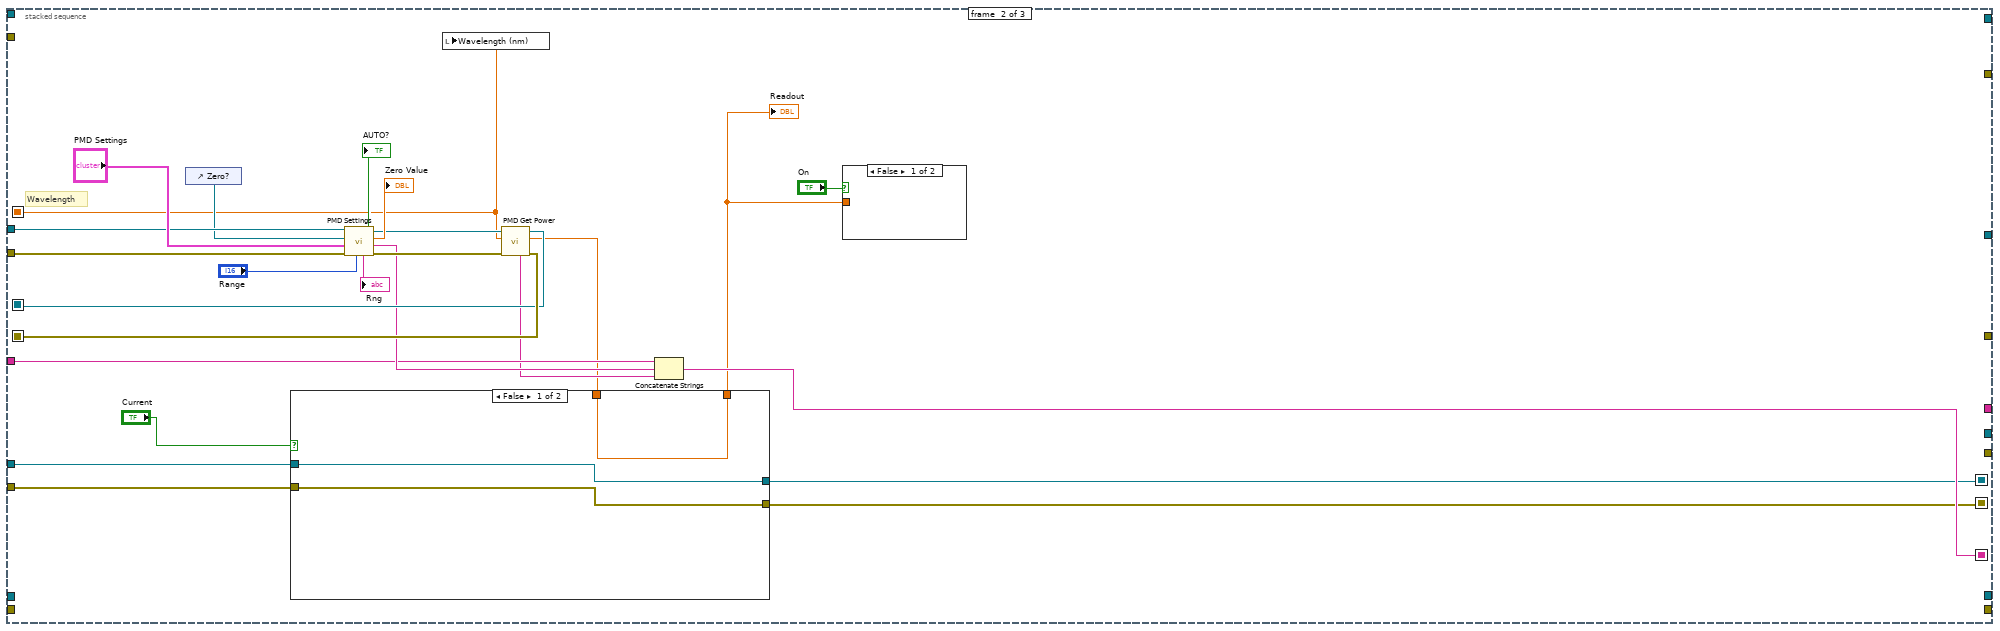
[diagram p12: hidden frame]
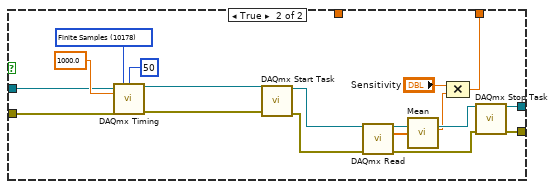
[diagram p13: hidden frame]
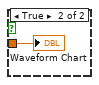
[diagram p14: hidden frame]
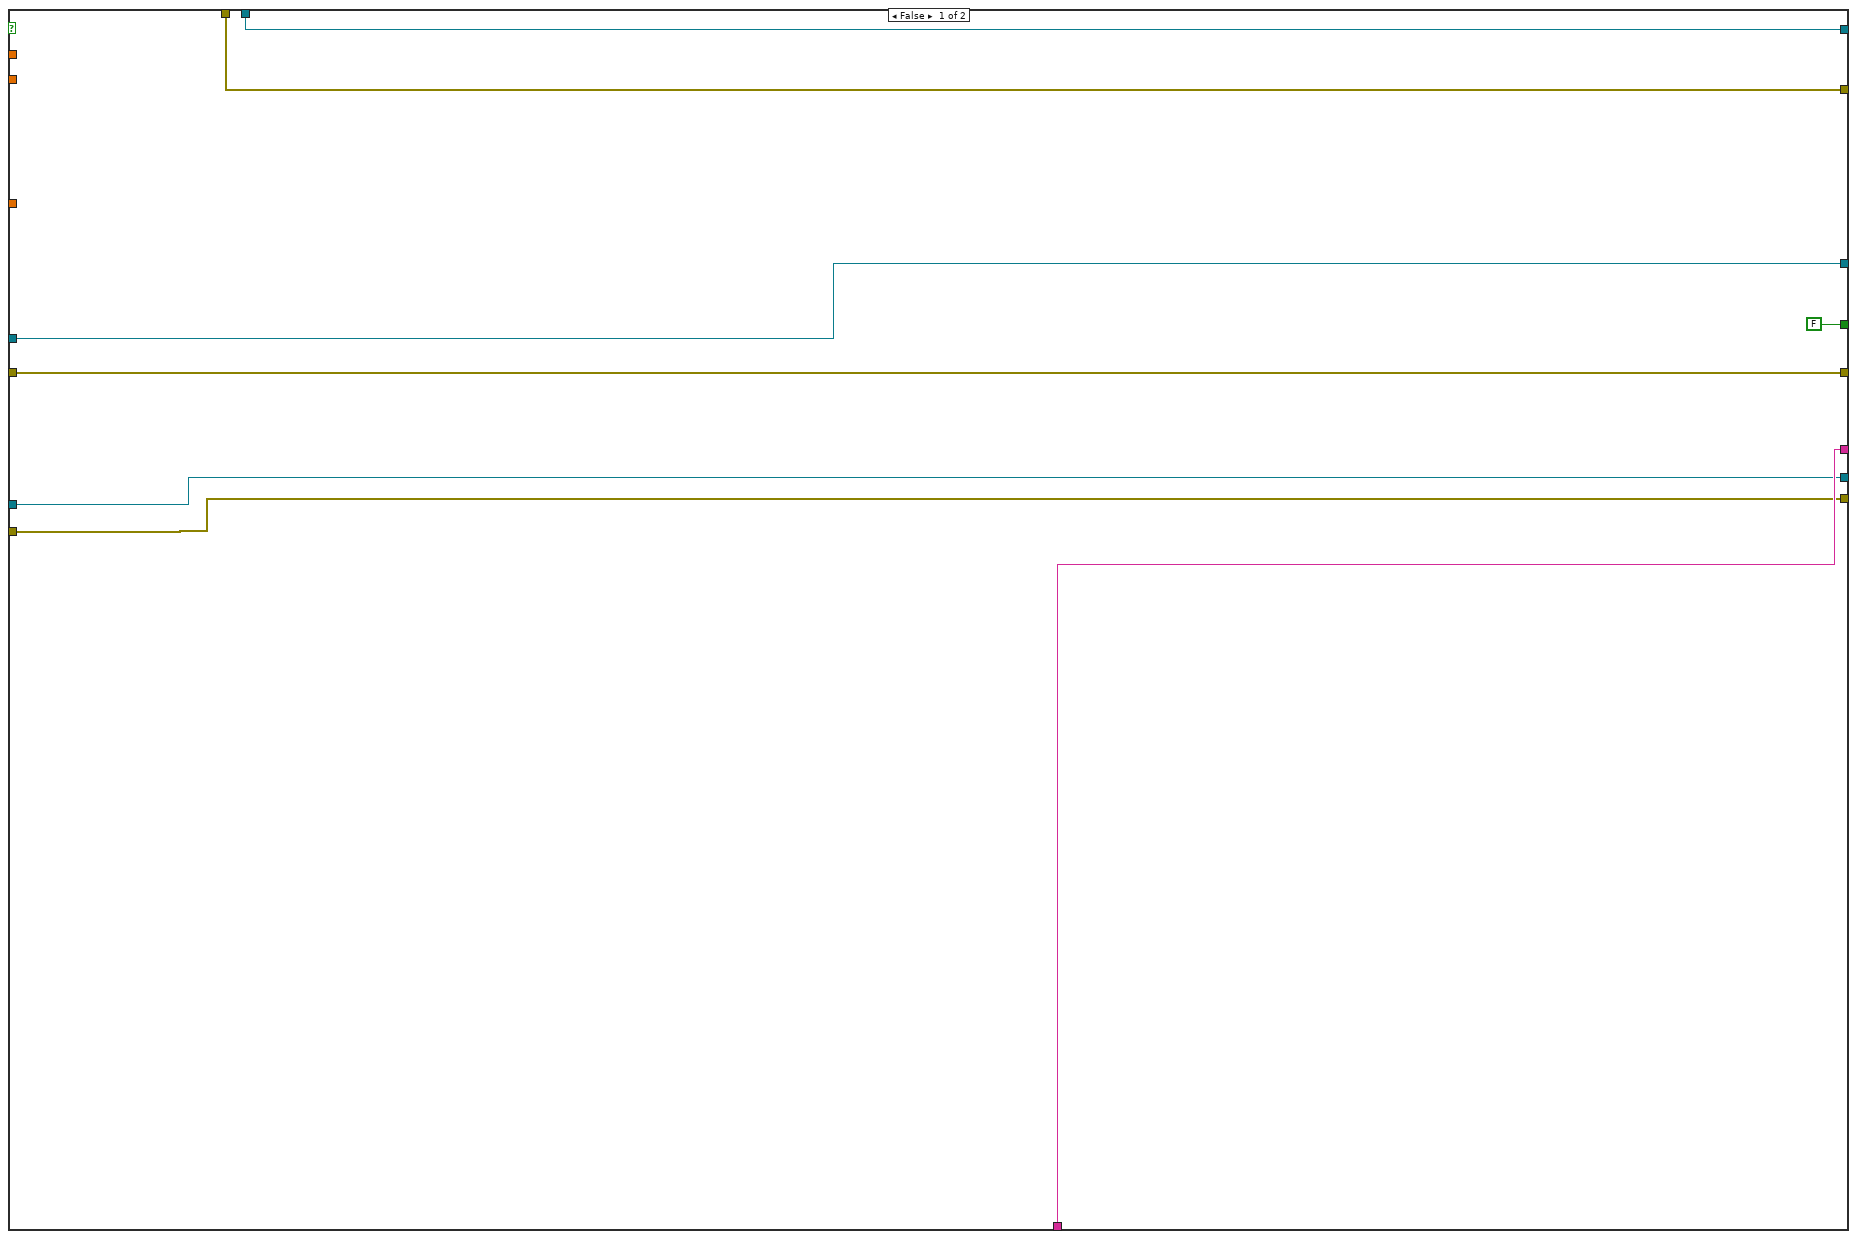
[diagram p15: hidden frame]
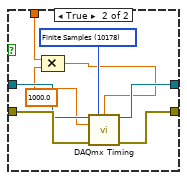
[diagram p16: hidden frame]
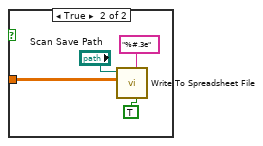
[diagram p17: hidden frame]
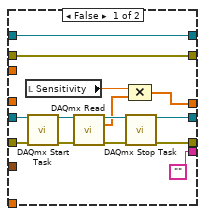
[diagram p18: hidden frame]
diagram:
  n1 = flat-sequence {
    tunnel: [w39] -> w20
    tunnel: [w38] -> w19
    tunnel: [w37] -> w18
    tunnel: [w36] -> w17
    tunnel: [w23] -> w12
    tunnel: [w24] -> w9
    tunnel: [w29] -> w8
    tunnel: [w30] -> w7
    tunnel: [w28] -> w6
    tunnel: [w27] -> w5
    tunnel: w20 -> [w64]
    tunnel: w19 -> [w65]
    tunnel: w18 -> [w63]
    tunnel: w17 -> [w62]
    tunnel: [w61] -> w16
    tunnel: [w60] -> w15
    tunnel: [w59] -> w14
    tunnel: [w58] -> w13
    tunnel: w12 -> [w55]
    tunnel: [w46] -> w11
    tunnel: [w45] -> w10
    tunnel: w9 -> [w56]
    tunnel: w8 -> [w54]
    tunnel: w7 -> [w53]
    tunnel: w6 -> [w52]
    tunnel: w5 -> [w51]
    tunnel: [w47] -> w4
    tunnel: [w48] -> w3
    tunnel: [w49] -> w2
    tunnel: [w50] -> w1
    tunnel: w16 -> [w526]
    tunnel: w15 -> [w525]
    tunnel: w14 -> [w524]
    tunnel: w13 -> [w523]
    tunnel: w11 -> [w521]
    tunnel: w10 -> [w522]
    tunnel: w4 -> [w520]
    tunnel: w3 -> [w519]
    tunnel: w2 -> [w518]
    tunnel: w1 -> [w517]
    frame #0 {
      w25 = -10.0 ("minimum value")
      w26 = 10.0 ("maximum value")
      n2 = call "PM100D_Initialize.vi"() -> ("error out"=w43:errorcluster, "Instrument"=→"IDN String":string, "VISA out"=w44:refnum<visa-resource-name>)  [unwired: 2 in, 1 out]
      n3 = call-poly <vilib>:"DAQmx Create Virtual Channel.vi"("maximum value"=w26, "minimum value"=w25, "physical channels"="Output A") -> ("task out"=w30:refnum<k21>, "error out"=w29:errorcluster)  [unwired: 11 in]
      n4 = call-poly <vilib>:"DAQmx Create Virtual Channel.vi"("maximum value"=10.0, "minimum value"=-10.0, "physical channels"="Input Channel") -> ("task out"=w24:refnum<k21>, "error out"=w23:errorcluster)  [unwired: 11 in]
      n5 = call "PM100D_SensorFlag.vi"("error in (no error)"=w43, "VISA in"=w44) -> ("error out"=w39:errorcluster, "VISA out"=w38:refnum<visa-resource-name>, "sn"=→"Sensor SN":string, "name"=→"Sensor Name":string)  [unwired: 2 in, 4 out]
      n6 = call-poly <vilib>:"DAQmx Create Virtual Channel.vi"("maximum value"=w26, "minimum value"=w25, "physical channels"="Output B") -> ("task out"=w27:refnum<k21>, "error out"=w28:errorcluster)  [unwired: 11 in]
      n7 = call "OpenMono.vi"("Mono Port"="Mono Port") -> ("VISA resource name out"=w37:refnum<visa-resource-name>, "error out"=w36:errorcluster)
      "Busy" <- FALSE ("Busy")
    }
    frame #1 {
      n8 = while {
        tunnel: w65 -> [w86]
        tunnel: w63 -> [w88]
        tunnel: [w83] -> w60
        tunnel: [w81] -> w58
        shift-right: [w80] -> w59
        shift-left: w64 -> [w85]
        shift-right: [w82] -> w61
        shift-left: w62 -> [w87]
        shift-right: [w78] -> _
        shift-left: "" -> [w79]
        shift-right: [w67] -> w45
        shift-left: w55 -> [w76]
        shift-right: [w66] -> w46
        shift-left: w56 -> [w77]
        shift-right: [w68] -> w50
        shift-left: w53 -> [w75]
        shift-right: [w69] -> w49
        shift-left: w54 -> [w74]
        shift-right: [w70] -> w48
        shift-left: w51 -> [w72]
        shift-right: [w71] -> w47
        shift-left: w52 -> [w73]
        stop <- "Exit" stop-if-true
        n9 = stacked-sequence {
          seq-local: [w107 _ _] -> [_ w203 _]
          seq-local: [w112 _ _] -> [_ _ w256]
          seq-local: [w111 _ _] -> [_ _ w255]
          seq-local: [_ w210 _] -> [_ _ w254]
          seq-local: [_ w211 _] -> [_ _ w253]
          seq-local: [_ w204 _] -> [_ _ w247]
          seq-local: [_ w198 _] -> [_ _ w243]
          seq-local: [_ w199 _] -> [_ _ w242]
          tunnel: w88 -> [w118 _ _]
          tunnel: w87 -> [w117 _ _]
          tunnel: w86 -> [_ w213 _]
          tunnel: w85 -> [_ w212 _]
          tunnel: [_ _ w252] -> w83
          tunnel: [_ _ w251] -> w82
          tunnel: [_ _ w250] -> w81
          tunnel: [_ _ w249] -> w80
          tunnel: w79 -> [_ w206 _]
          tunnel: [_ _ w246] -> w78
          tunnel: w77 -> [_ w197 _]
          tunnel: w76 -> [_ w196 _]
          tunnel: [_ _ w245] -> w66
          tunnel: [_ _ w244] -> w67
          tunnel: w75 -> [w102 _ _]
          tunnel: w74 -> [w103 _ _]
          tunnel: w73 -> [w105 _ _]
          tunnel: w72 -> [w104 _ _]
          tunnel: [w101 _ _] -> w71
          tunnel: [w100 _ _] -> w70
          tunnel: [w99 _ _] -> w69
          tunnel: [w98 _ _] -> w68
          frame #0 {
            # "Wavelength"
            n10 = while {
              shift-right: [w140] -> w89
              shift-left: _ -> [w139]
              tunnel: "Voltage B" -> [w140]
              tunnel: [w139] -> w94
              tunnel: "Voltage A" -> [w138]
              shift-right: [w138] -> w90
              shift-left: _ -> [w137]
              tunnel: [w137] -> w95
              stop <- TRUE stop-if-true
            }
            n11 = case shown="False" "Send Question" {
              tunnel: w118 -> [w188 w194]
              tunnel: w117 -> [w187 w193]
              tunnel: [w188 w192] -> w120
              tunnel: [w187 w191] -> w119
              frame False {
                (unwired) FALSE ("Read Error")
              }
              frame True {
                n12 = control-ref of="Busy"() -> (w189:refnum<vi>)
                n13 = call "ReadMono.vi"("Busy"=w189, "error in (no error)"=w193, "Cmd"="Ask?", "Mono Port"=w194) -> ("error out"=w191:errorcluster, "Response"=→"Reply":string, "Mono Port Out"=w192:refnum<visa-resource-name>)  [unwired: 2 in, 1 out]
              }
            }
            n14 = Not Equal?(x=w90, y=w95) -> (x != y?=w93:bool)
            n15 = Not Equal?(x=w89, y=w94) -> (x != y?=w92:bool)
            n16 = Or(x=w93, y=w92) -> (x .or. y?=w91:bool)
            n17 = case shown="False" w91 {
              tunnel: w105 -> [w123 w136]
              tunnel: w104 -> [w124 w135]
              tunnel: w103 -> [w125 w134]
              tunnel: w102 -> [w126 w133]
              tunnel: [w123 w132] -> w101
              tunnel: [w124 w131] -> w100
              tunnel: [w125 w130] -> w99
              tunnel: [w126 w129] -> w98
              tunnel: w90 -> [_ w127]
              tunnel: w89 -> [_ w128]
              frame False {
              }
              frame True {
                n18 = call-poly <vilib>:"DAQmx Write.vi"("task/channels in"=w135, "data"=w128, "error in"=w136) -> ("task out"=w131:refnum<k21>, "error out"=w132:errorcluster)  [unwired: 10 in, 1 out]
                n19 = call-poly <vilib>:"DAQmx Write.vi"("task/channels in"=w133, "data"=w127, "error in"=w134) -> ("task out"=w129:refnum<k21>, "error out"=w130:errorcluster)  [unwired: 10 in, 1 out]
              }
            }
            n20 = case shown="False" "Send Command" {
              tunnel: w120 -> [w173 w186]
              tunnel: w119 -> [w172 w185]
              tunnel: [w173 w178] -> w115
              tunnel: [w172 w177] -> w114
              tunnel: "Wavelength (nm)" -> [w171 w181]
              tunnel: [w171 w181] -> w113
              frame False {
              }
              frame True {
                w176 = u16 0 items=["?nm", "?nm/min", "?grating", "?turret", "?gratings"] ("Cmd")
                n21 = control-ref of="Busy"() -> (w174:refnum<vi>)
                n22 = call "CmdMono.vi"("Busy"=w174, "Scan Speed (nm/min)"="Scan Speed (nm/min)", "error in (no error)"=w185, "Wavelength (nm)"=w181, "Cmd"="Command", "Mono Port"=w186) -> ("error out"=w179:errorcluster, "Response"=→"Done?":string, "Mono Port Out"=w180:refnum<visa-resource-name>)  [unwired: 2 in, 1 out]
                n23 = call "ReadMono.vi"("Busy"=w174, "error in (no error)"=w179, "Cmd"=w176, "Mono Port"=w180) -> ("error out"=w177:errorcluster, "Response"=w175:string, "Mono Port Out"=w178:refnum<visa-resource-name>)  [unwired: 2 in, 1 out]
                n24 = local write "Reply"(w175) -> ()
              }
            }
            n25 = case shown="False" "Step" {
              tunnel: w115 -> [w151 w170]
              tunnel: w114 -> [w150 w169]
              tunnel: w113 -> [w149 w163]
              tunnel: [w151 w156] -> w112
              tunnel: [w150 w157] -> w111
              tunnel: "Increment (nm)" -> [_ w162]
              tunnel: [w149 w152] -> w107
              frame False {
              }
              frame True {
                w154 = u16 0 items=["?nm", "?nm/min", "?grating", "?turret", "?gratings"] ("Cmd")
                w161 = u16 1 items=["nm", "goto", "nm/min", "VIS grating", "IR grating"] ("Cmd")
                n26 = Select(t=1, s="Up", f=-1) -> (s? t:f=w168:i32)
                n27 = control-ref of="Busy"() -> (w153:refnum<vi>)
                n28 = Compound Arithmetic op=MULTIPLY(w168, w162) -> (w164:dbl)
                n29 = Compound Arithmetic op=ADD(w164, w163) -> (w152:dbl)
                n30 = call "CmdMono.vi"("Busy"=w153, "error in (no error)"=w169, "Wavelength (nm)"=w152, "Cmd"=w161, "Mono Port"=w170) -> ("error out"=w158:errorcluster, "Response"=w160:string, "Mono Port Out"=w159:refnum<visa-resource-name>)  [unwired: 3 in, 1 out]
                n31 = call "ReadMono.vi"("Busy"=w153, "error in (no error)"=w158, "Cmd"=w154, "Mono Port"=w159) -> ("error out"=w157:errorcluster, "Response"=w155:string, "Mono Port Out"=w156:refnum<visa-resource-name>)  [unwired: 2 in, 1 out]
                n32 = local write "Done?"(w160) -> ()
                n33 = local write "Reply"(w155) -> ()
              }
            }
            n34 = event shown="[0] Timeout" {
              selector: _ -> [_ _]
              dyn-events: _ -> [_ _]
              timeout: 0 -> [_ _]
              event Timeout {
                n35 = event-data() -> ()  [unwired: 1 in, 2 out]
              }
              event "Send Command", "Step": Mouse Up {
                n36 = event-data() -> ()  [unwired: 1 in, 1 out]
                n37 = local write "Done?"("   ..." ("Done?")) -> ()
              }
            }
            n38 = event shown="[0] Timeout" {
              selector: _ -> [_ _ _]
              dyn-events: _ -> [_ _ _]
              timeout: 0 -> [_ _ _]
              event Timeout {
                n39 = event-data() -> ()  [unwired: 1 in, 2 out]
              }
              event "Power": Mouse Down? {
                n40 = event-data() -> ()  [unwired: 1 in, 7 out]
                n41 = local read "Power"() -> (w142:bool)
                n42 = case shown="False" w142 {
                  selector: w142 -> [w144 _]
                  frame False {
                    w143 = "Power (W)" ("Y Scale.Name Label.Text")
                    n43 = local write "Current"(w144) -> ()
                    n44 = property on="ScanGraph" class="XYGraph (strict)"("YScale.NameLbl.Text"=w143) -> ()  [unwired: 2 in, 2 out]
                    n45 = property on="Waveform Chart" class="WFChart (strict)"("YScale.NameLbl.Text"=w143) -> ()  [unwired: 2 in, 2 out]
                  }
                  frame True {
                  }
                }
                n46 = event-data("Discard?"=w142) -> ()  [unwired: 1 in, 1 out]
              }
              event "Current": Mouse Down? {
                n47 = event-data() -> ()  [unwired: 1 in, 7 out]
                n48 = local read "Current"() -> (w145:bool)
                n49 = case shown="False" w145 {
                  selector: w145 -> [w146 _]
                  frame False {
                    w147 = "Current (A)" ("Y Scale.Name Label.Text")
                    n50 = local write "Power"(w146) -> ()
                    n51 = property on="ScanGraph" class="XYGraph (strict)"("YScale.NameLbl.Text"=w147) -> ()  [unwired: 2 in, 2 out]
                    n52 = property on="Waveform Chart" class="WFChart (strict)"("YScale.NameLbl.Text"=w147) -> ()  [unwired: 2 in, 2 out]
                  }
                  frame True {
                  }
                }
                n53 = event-data("Discard?"=w145) -> ()  [unwired: 1 in, 1 out]
              }
            }
          }
          frame #1 {
            # "Wavelength"
            n54 = control-ref of="Zero?"() -> (w208:refnum<vi>)
            n55 = call "PMD Settings.vi"("Visa In"=w213, "Zero?"=w208, "PMD Settings In"="PMD Settings", "Error In"=w212, "Range"="Range") -> ("AUTO?"=→"AUTO?":bool, "Rng"=→"Rng":string, "Visa Out"=w216:refnum<visa-resource-name>, "ZeroValue"=→"Zero Value":dbl, "PM Error log"=w207:string, "error out"=w215:errorcluster)
            n56 = local write "Wavelength (nm)"(w203) -> ()
            n57 = call "PMD Get Power.vi"("VISA In"=w216, "Wavelength (nm)"=w203, "error in"=w215) -> ("PMD Error"=w205:string, "VISA out"=w210:refnum<visa-resource-name>, "Readout value"=w202:dbl, "error out"=w211:errorcluster)  [unwired: 1 in, 2 out]
            n58 = case shown="False" "Current" {
              tunnel: w202 -> [w223 _]
              tunnel: w197 -> [w222 w226]
              tunnel: w196 -> [w221 w227]
              tunnel: [w223 w239] -> w200
              tunnel: [w221 w235] -> w198
              tunnel: [w222 w236] -> w199
              frame False {
              }
              frame True {
                w229 = 10178 items=["Finite Samples"=10178, "Continuous Samples"=10123, "Hardware Timed Single Point"=12522] ("sample mode")
                n59 = call-poly <vilib>:"DAQmx Timing.vi"("task/channels in"=w226, "sample mode"=w229, "samples per channel"=50, "rate"=1000.0, "error in"=w227) -> ("task out"=w225:refnum<k21>, "error out"=w224:errorcluster)  [unwired: 9 in]
                n60 = call <vilib>:"DAQmx Start Task.vi"("task/channels in"=w225, "error in"=w224) -> ("task out"=w237:refnum<k21>, "error out"=w238:errorcluster)  [unwired: 12 in]
                n61 = call-poly <vilib>:"DAQmx Read.vi"("task/channels in"=w237, "error in"=w238) -> ("task out"=w233:refnum<k21>, "data"=w232:dbl[], "error out"=w234:errorcluster)  [unwired: 11 in]
                n62 = call <vilib>:"Mean.vi"("X"=w232) -> ("mean"=w231:dbl)  [unwired: 1 out]
                n63 = Compound Arithmetic op=MULTIPLY("Sensitivity", w231) -> (w239:dbl)
                n64 = call <vilib>:"DAQmx Stop Task.vi"("task/channels in"=w233, "error in"=w234) -> ("task out"=w236:refnum<k21>, "error out"=w235:errorcluster)  [unwired: 12 in]
              }
            }
            "Readout" <- w200
            n65 = Concatenate Strings(w206, w207, w205) -> (w204:string)
            n66 = case shown="False" "On" {
              tunnel: w200 -> [_ w241]
              frame False {
              }
              frame True {
                "Waveform Chart" <- w241
              }
            }
          }
          frame #2 {
            # "Wavelength"
            n67 = Subtract(x="End", y="Start") -> (x-y=w261:dbl)
            n68 = Divide(x=w261, y="Step Size (nm)") -> (x/y=w260:dbl)
            n69 = Round To Nearest(number=w260) -> (nearest integer value=w259:dbl)
            n70 = case shown="True" "Scan" {
              tunnel: w259 -> [_ w326]
              tunnel: w255 -> [w269 w328]
              tunnel: w256 -> [w268 w329]
              tunnel: "Start" -> [_ w331]
              tunnel: "Step Size (nm)" -> [_ w330]
              tunnel: w254 -> [w271 w324]
              tunnel: w253 -> [w270 w323]
              tunnel: [w271 w312] -> w250
              tunnel: [w270 w322] -> w249
              tunnel: [w269 w321] -> w251
              tunnel: [w268 w320] -> w252
              tunnel: [FALSE ("Scan") FALSE ("Scan")] -> w248
              tunnel: w247 -> [w266 w314]
              tunnel: [w266 w313] -> w246
              tunnel: [w265 w311] -> w245
              tunnel: [w264 w310] -> w244
              tunnel: w243 -> [w264 w308]
              tunnel: w242 -> [w265 w307]
              frame False {
              }
              frame True {
                w283 = 10178 items=["Finite Samples"=10178, "Continuous Samples"=10123, "Hardware Timed Single Point"=12522] ("sample mode")
                w327 = dbl[] []
                # "Read Inital values"
                # "Setup inputs/outputs"
                n71 = call-poly <vilib>:"DAQmx Create Virtual Channel.vi"("maximum value"=4.0, "minimum value"=-4.0, "physical channels"="Scan mirrors out") -> ("task out"=w291:refnum<k21>, "error out"=w290:errorcluster)  [unwired: 11 in]
                n72 = call-poly <vilib>:"DAQmx Create Virtual Channel.vi"("maximum value"=10.0, "minimum value"=-10.0, "physical channels"="Scan Mirrors in") -> ("task out"=w298:refnum<k21>, "error out"=w302:errorcluster)  [unwired: 11 in]
                n73 = local read "Current"() -> (w309:bool)
                n74 = case shown="False" w309 {
                  tunnel: w308 -> [w332 w340]
                  tunnel: w307 -> [w333 w339]
                  tunnel: [w333 w338] -> w306
                  tunnel: [w332 w337] -> w305
                  tunnel: "Step Time (sec)" -> [_ w336]
                  frame False {
                  }
                  frame True {
                    w341 = 10178 items=["Finite Samples"=10178, "Continuous Samples"=10123, "Hardware Timed Single Point"=12522] ("sample mode")
                    w335 = 1000.0 ("rate")
                    n75 = Compound Arithmetic op=MULTIPLY(w336, w335) -> (w334:dbl)
                    n76 = call-poly <vilib>:"DAQmx Timing.vi"("task/channels in"=w339, "sample mode"=w341, "samples per channel"=w334, "rate"=w335, "error in"=w340) -> ("task out"=w338:refnum<k21>, "error out"=w337:errorcluster)  [unwired: 9 in]
                  }
                }
                n77 = call-poly <vilib>:"DAQmx Timing.vi"("task/channels in"=w291, "sample mode"=w283, "samples per channel"=1000, "rate"=1250.0, "error in"=w290) -> ("task out"=w280:refnum<k21>, "error out"=w281:errorcluster)  [unwired: 9 in]
                n78 = call-poly <vilib>:"DAQmx Read.vi"("task/channels in"=w298, "timeout"=10.0, "error in"=w302) -> ("task out"=w289:refnum<k21>, "data"=w297:dbl[], "error out"=w288:errorcluster)  [unwired: 10 in]
                n79 = Increment(x=w326) -> (x+1=w325:dbl)
                n80 = Index Array(array=w297, index=0) -> (element=w274:dbl)
                n81 = Index Array(array=w297, index=1) -> (element=w276:dbl)
                n82 = Add(x=w276, y=0.0067) -> (x+y=w275:dbl)
                n83 = Add(x=w274, y=0.0055) -> (x+y=w272:dbl)
                n84 = for {
                  N: w325 -> [_]
                  tunnel: w329 -> [w431]
                  tunnel: w331 -> [w427]
                  tunnel: w330 -> [w429]
                  shift-right: [w415] -> w319
                  shift-left: w327 -> [w433]
                  shift-right: [w426] -> w321
                  shift-left: w328 -> [w432]
                  shift-right: [w412] -> w318
                  shift-left: w327 -> [w413]
                  tunnel: w324 -> [w424]
                  shift-right: [w419] -> w322
                  shift-left: w323 -> [w423]
                  tunnel: [w418] -> w312
                  tunnel: [w417] -> w320
                  shift-right: [w410] -> w313
                  shift-left: w314 -> [w411]
                  shift-right: [w407] -> w310
                  shift-left: w305 -> [w402]
                  shift-right: [w406] -> w311
                  shift-left: w306 -> [w403]
                  tunnel: "Step Time (sec)" -> [w404]
                  tunnel: w272 -> [w356]
                  tunnel: w275 -> [w357]
                  shift-right: [w386] -> w278
                  shift-left: w281 -> [w384]
                  shift-right: [w376] -> w287
                  shift-left: w289 -> [w397]
                  shift-right: [w377] -> w286
                  shift-left: w288 -> [w396]
                  tunnel: "Volts/pixel" -> [w393]
                  tunnel: w280 -> [w385]
                  tunnel: [w346] -> w279
                  i -> [w430]
                  stop <- "STOP" stop-if-true
                  # "Move sm to correct positino"
                  # "Monitor array being sent to write"
                  # "Read after writing"
                  # "Calculate correction"
                  # "Correct for AO/AI offset"
                  # "Read current location"
                  n85 = Compound Arithmetic op=MULTIPLY(w429, w430) -> (w428:dbl)
                  n86 = Compound Arithmetic op=ADD(w427, w428) -> (w395:dbl)
                  n87 = local write "Wavelength (nm)"(w395) -> ()
                  n88 = call-poly <vilib>:"DAQmx Read.vi"("task/channels in"=w397, "error in"=w396) -> ("task out"=w351:refnum<k21>, "data"=w398:dbl[], "error out"=w378:errorcluster)  [unwired: 11 in]
                  n89 = flat-sequence {
                    tunnel: w432 -> [w454]
                    tunnel: w431 -> [w453]
                    tunnel: w395 -> [w449]
                    tunnel: [w438] -> w426
                    tunnel: w424 -> [w451]
                    tunnel: w423 -> [w450]
                    tunnel: [w451] -> w422
                    tunnel: [w450] -> w421
                    tunnel: [w449] -> w420
                    tunnel: [w443] -> w417
                    tunnel: [w439] -> w414
                    tunnel: w402 -> [w436]
                    tunnel: [w437] -> w409
                    tunnel: w403 -> [w437]
                    tunnel: [w436] -> w408
                    tunnel: [w435] -> w405
                    tunnel: w404 -> [w435]
                    tunnel: w351 -> [w434]
                    tunnel: [w434] -> w350
                    tunnel: [w470] -> w401
                    tunnel: w422 -> [w469]
                    tunnel: w421 -> [w468]
                    tunnel: w420 -> [w467]
                    tunnel: [w463] -> w419
                    tunnel: [w466] -> w418
                    tunnel: w411 -> [w465]
                    tunnel: [w464] -> w410
                    tunnel: w409 -> [w461]
                    tunnel: w408 -> [w460]
                    tunnel: [w458] -> w406
                    tunnel: [w459] -> w407
                    tunnel: w405 -> [w462]
                    tunnel: w348 -> [w456]
                    tunnel: [w456] -> w347
                    tunnel: [w455] -> w349
                    tunnel: w350 -> [w455]
                    frame #0 {
                      w445 = u16 0 items=["?nm", "?nm/min", "?grating", "?turret", "?gratings"] ("Cmd")
                      w452 = u16 1 items=["nm", "goto", "nm/min", "VIS grating", "IR grating"] ("Cmd")
                      n90 = control-ref of="Busy"() -> (w444:refnum<vi>)
                      n91 = call "CmdMono.vi"("Busy"=w444, "error in (no error)"=w454, "Wavelength (nm)"=w449, "Cmd"=w452, "Mono Port"=w453) -> ("error out"=w446:errorcluster, "Response"=w448:string, "Mono Port Out"=w447:refnum<visa-resource-name>)  [unwired: 3 in, 1 out]
                      n92 = local write "Done?"(w448) -> ()
                      n93 = call "ReadMono.vi"("Busy"=w444, "error in (no error)"=w446, "Cmd"=w445, "Mono Port"=w447) -> ("error out"=w438:errorcluster, "Response"=w441:string, "Mono Port Out"=w443:refnum<visa-resource-name>)  [unwired: 2 in, 1 out]
                      n94 = Match Pattern(string=w441, regular expression=" nm") -> (before substring=w440:string)  [unwired: 1 in, 3 out]
                      n95 = Fract/Exp String To Number(string=w440) -> (number=w439:dbl)  [unwired: 3 in, 1 out]
                      n96 = local write "Reply"(w441) -> ()
                    }
                    frame #1 {
                      n97 = Get Date/Time In Seconds() -> (seconds since 1Jan1904=w472:timestamp)
                      n98 = case shown="True" "Power" {
                        tunnel: dbl[] [] -> [_ w500]
                        tunnel: w472 -> [_ w499]
                        tunnel: [w474 w498] -> w471
                        tunnel: w469 -> [w486 w497]
                        tunnel: w468 -> [w485 w496]
                        tunnel: w467 -> [_ w495]
                        tunnel: [w486 w494] -> w466
                        tunnel: w465 -> [_ w493]
                        tunnel: ["" w492] -> w464
                        tunnel: [w485 w491] -> w463
                        tunnel: w462 -> [_ w490]
                        tunnel: w461 -> [w484 w488]
                        tunnel: w460 -> [w483 w489]
                        tunnel: [w478 w489] -> w459
                        tunnel: [w477 w488] -> w458
                        frame False {
                          n99 = local read "Sensitivity"() -> (w475:dbl)
                          n100 = call <vilib>:"DAQmx Start Task.vi"("task/channels in"=w484, "error in"=w483) -> ("task out"=w482:refnum<k21>, "error out"=w481:errorcluster)  [unwired: 12 in]
                          n101 = call-poly <vilib>:"DAQmx Read.vi"("task/channels in"=w482, "error in"=w481) -> ("task out"=w480:refnum<k21>, "data"=w476:dbl[], "error out"=w479:errorcluster)  [unwired: 11 in]
                          n102 = call <vilib>:"DAQmx Stop Task.vi"("task/channels in"=w480, "error in"=w479) -> ("task out"=w477:refnum<k21>, "error out"=w478:errorcluster)  [unwired: 12 in]
                          n103 = Compound Arithmetic op=MULTIPLY(w475, w476) -> (w474:dbl[])
                        }
                        frame True {
                          n104 = while {
                            shift-right: [w515] -> w498
                            shift-left: w500 -> [w516]
                            tunnel: w499 -> [w513]
                            tunnel: w497 -> [w508]
                            tunnel: w495 -> [w504]
                            tunnel: [w506] -> w494
                            tunnel: w493 -> [w510]
                            tunnel: [w509] -> w492
                            shift-right: [w502] -> w491
                            shift-left: w496 -> [w507]
                            tunnel: w490 -> [w501]
                            stop <- w511 stop-if-true
                            n105 = Get Date/Time In Seconds() -> (seconds since 1Jan1904=w514:timestamp)
                            n106 = Subtract(x=w514, y=w513) -> (x-y=w512:dbl)
                            n107 = call "PMD Get Power.vi"("VISA In"=w508, "Wavelength (nm)"=w504, "error in"=w507) -> ("PMD Error"=w503:string, "VISA out"=w506:refnum<visa-resource-name>, "Readout value"=w505:dbl, "error out"=w502:errorcluster)  [unwired: 1 in, 2 out]
                            n108 = Greater Or Equal?(x=w512, y=w501) -> (x >= y?=w511:bool)
                            n109 = Build Array (concatenate)(w516, w505) -> (w515:dbl[])
                            n110 = Concatenate Strings(w510, w503) -> (w509:string)
                          }
                        }
                      }
                      n111 = call <vilib>:"Mean.vi"("X"=w471) -> ("mean"=w470:dbl)  [unwired: 1 out]
                    }
                  }
                  n112 = Index Array(array=w398, index=0) -> (element=w369:dbl)
                  n113 = Index Array(array=w398, index=1) -> (element=w366:dbl)
                  n114 = Add(x=0.0067, y=w366) -> (x+y=w364:dbl)
                  "Yin" <- w364
                  n115 = Add(x=0.0055, y=w369) -> (x+y=w367:dbl)
                  "Xin" <- w367
                  n116 = Build Array (concatenate)(w413, w414) -> (w412:dbl[])
                  n117 = call "SM correction ver2.vi"("V in x"=w367, "nm in"=w395, "V in y"=w364, "V x initial"=w356, "Volts/pixel"=w393, "V y initial"=w357, "Array"="Correction") -> ("V out x"=w370:dbl[], "V out y"=w379:dbl[])
                  "Waveform Chart X" <- w370
                  "Waveform Chart  Y" <- w379
                  n118 = local write "Readout"(w401) -> ()
                  n119 = Build Array (concatenate)(w433, w401) -> (w415:dbl[])
                  n120 = call <vilib>:"DAQmx Start Task.vi"("task/channels in"=w385, "error in"=w384) -> ("task out"=w354:refnum<k21>, "error out"=w353:errorcluster)  [unwired: 12 in]
                  n121 = Build Array(w370, w379) -> (w372:dbl[][])
                  n122 = Bundle(w412, w415) -> (→"ScanGraph":cluster{dbl[], dbl[]})  [unwired: 1 in]
                  n123 = Negate(x=w372) -> (-x=w371:dbl[][])
                  n124 = call-poly <vilib>:"DAQmx Write.vi"("task/channels in"=w354, "auto start"=TRUE, "data"=w371, "timeout"=-1.0, "error in"=w353) -> ("task out"=w348:refnum<k21>, "number of samples written per channel"=→"number of samples written per channel":u32, "error out"=w355:errorcluster)  [unwired: 8 in]
                  n125 = local write "PM Error log"(w410) -> ()
                  n126 = Index Array(array=w370, index #1=0 ("index"), index #2=999 ("index")) -> (element #1=→"initial x":dbl, element #2=→"Final x":dbl)
                  n127 = Index Array(array=w379, index #1=0 ("index"), index #2=999 ("index")) -> (element #1=→"initial y":dbl, element #2=→"Final Y":dbl)
                  n128 = call-poly <vilib>:"DAQmx Read.vi"("task/channels in"=w349, "error in"=w378) -> ("task out"=w376:refnum<k21>, "data"=w373:dbl[], "error out"=w377:errorcluster)  [unwired: 11 in]
                  n129 = call <vilib>:"DAQmx Stop Task.vi"("task/channels in"=w347, "error in"=w355) -> ("task out"=w346:refnum<k21>, "error out"=w386:errorcluster)  [unwired: 12 in]
                  n130 = Index Array(array=w373, index=0) -> (element=w360:dbl)
                  n131 = Index Array(array=w373, index=1) -> (element=w361:dbl)
                  n132 = Add(x=0.0055, y=w360) -> (x+y=→"element":dbl)
                  n133 = Add(x=0.0067, y=w361) -> (x+y=→"element 2":dbl)
                }
                n134 = Build Array(w319, w318) -> (w317:dbl[][])
                n135 = call <vilib>:"DAQmx Stop Task.vi"("task/channels in"=w287, "error in"=w286) -> ()  [unwired: 12 in, 2 out]
                n136 = case shown="False" "Save" {
                  tunnel: w317 -> [_ w342]
                  frame False {
                  }
                  frame True {
                    n137 = call-poly <vilib>:"Write To Spreadsheet File.vi"("transpose? (no:F)"=TRUE, "format (%.3f)"="%#.3e", "2D data"=w342, "file path (dialog if empty)"="Scan Save Path") -> ()  [unwired: 4 in, 1 out]
                  }
                }
                n138 = call <vilib>:"DAQmx Clear Task.vi"("task in"=w279, "error in"=w278) -> ()  [unwired: 13 in, 1 out]
              }
            }
            n139 = local write "Scan"(w248) -> ()
          }
        }
        "PM Error log" <- w78
      }
    }
    frame #2 {
      n140 = call <vilib>:"DAQmx Clear Task.vi"("task in"=w521, "error in"=w522) -> ()  [unwired: 13 in, 1 out]
      n141 = call <vilib>:"DAQmx Clear Task.vi"("task in"=w517, "error in"=w518) -> ()  [unwired: 13 in, 1 out]
      n142 = call <vilib>:"DAQmx Clear Task.vi"("task in"=w519, "error in"=w520) -> ()  [unwired: 13 in, 1 out]
      n143 = VISA Close(VISA resource name=w525, error in (no error)=w526) -> (error out=w527:errorcluster)
      n144 = call "PM100D_Close.vi"("error in (no error)"=w524, "VISA resource name"=w523) -> ()  [unwired: 2 in]
      n145 = call <vilib>:"Simple Error Handler.vi"("error in (no error)"=w527) -> ()  [unwired: 1 in, 8 out]
    }
  }
